vi "main OP600_V2.vi"() -> ()   [LabVIEW 2020]
uses:
  SubVI/OP600ZP_state.ctl
  <userlib>/Alex.vi/FGV.ctl
  VG/VG_progressBar.vi
  SubVI/CheminDeBase.vi
  VG/PN.vi
  VG/PackType.vi
  VG/IS30%.vi
  SubVI/OP600ZP_VGConf.vi
  VG/Ubatt.vi
  VG/OCV.vi
panel:
  out "Revision":i32
  out "Progres":dbl(slide) scale=0.0..30.0
  out "IS30% ?":bool
  out "Cluster":T1
  out "VISA OUT":T2
  out "progression":u8(slide) scale=0.0..100.0
  out "PN":string
  out "errout 2":errorcluster={"status"=TRUE, "code"=0, "source"="PCAN_CHANNEL ILLEGAL"} caption="errout"
  out "errout":errorcluster caption="sortie d'erreur"
  out "STOP":bool
  out "TOP":string
  out "DRAW":picture
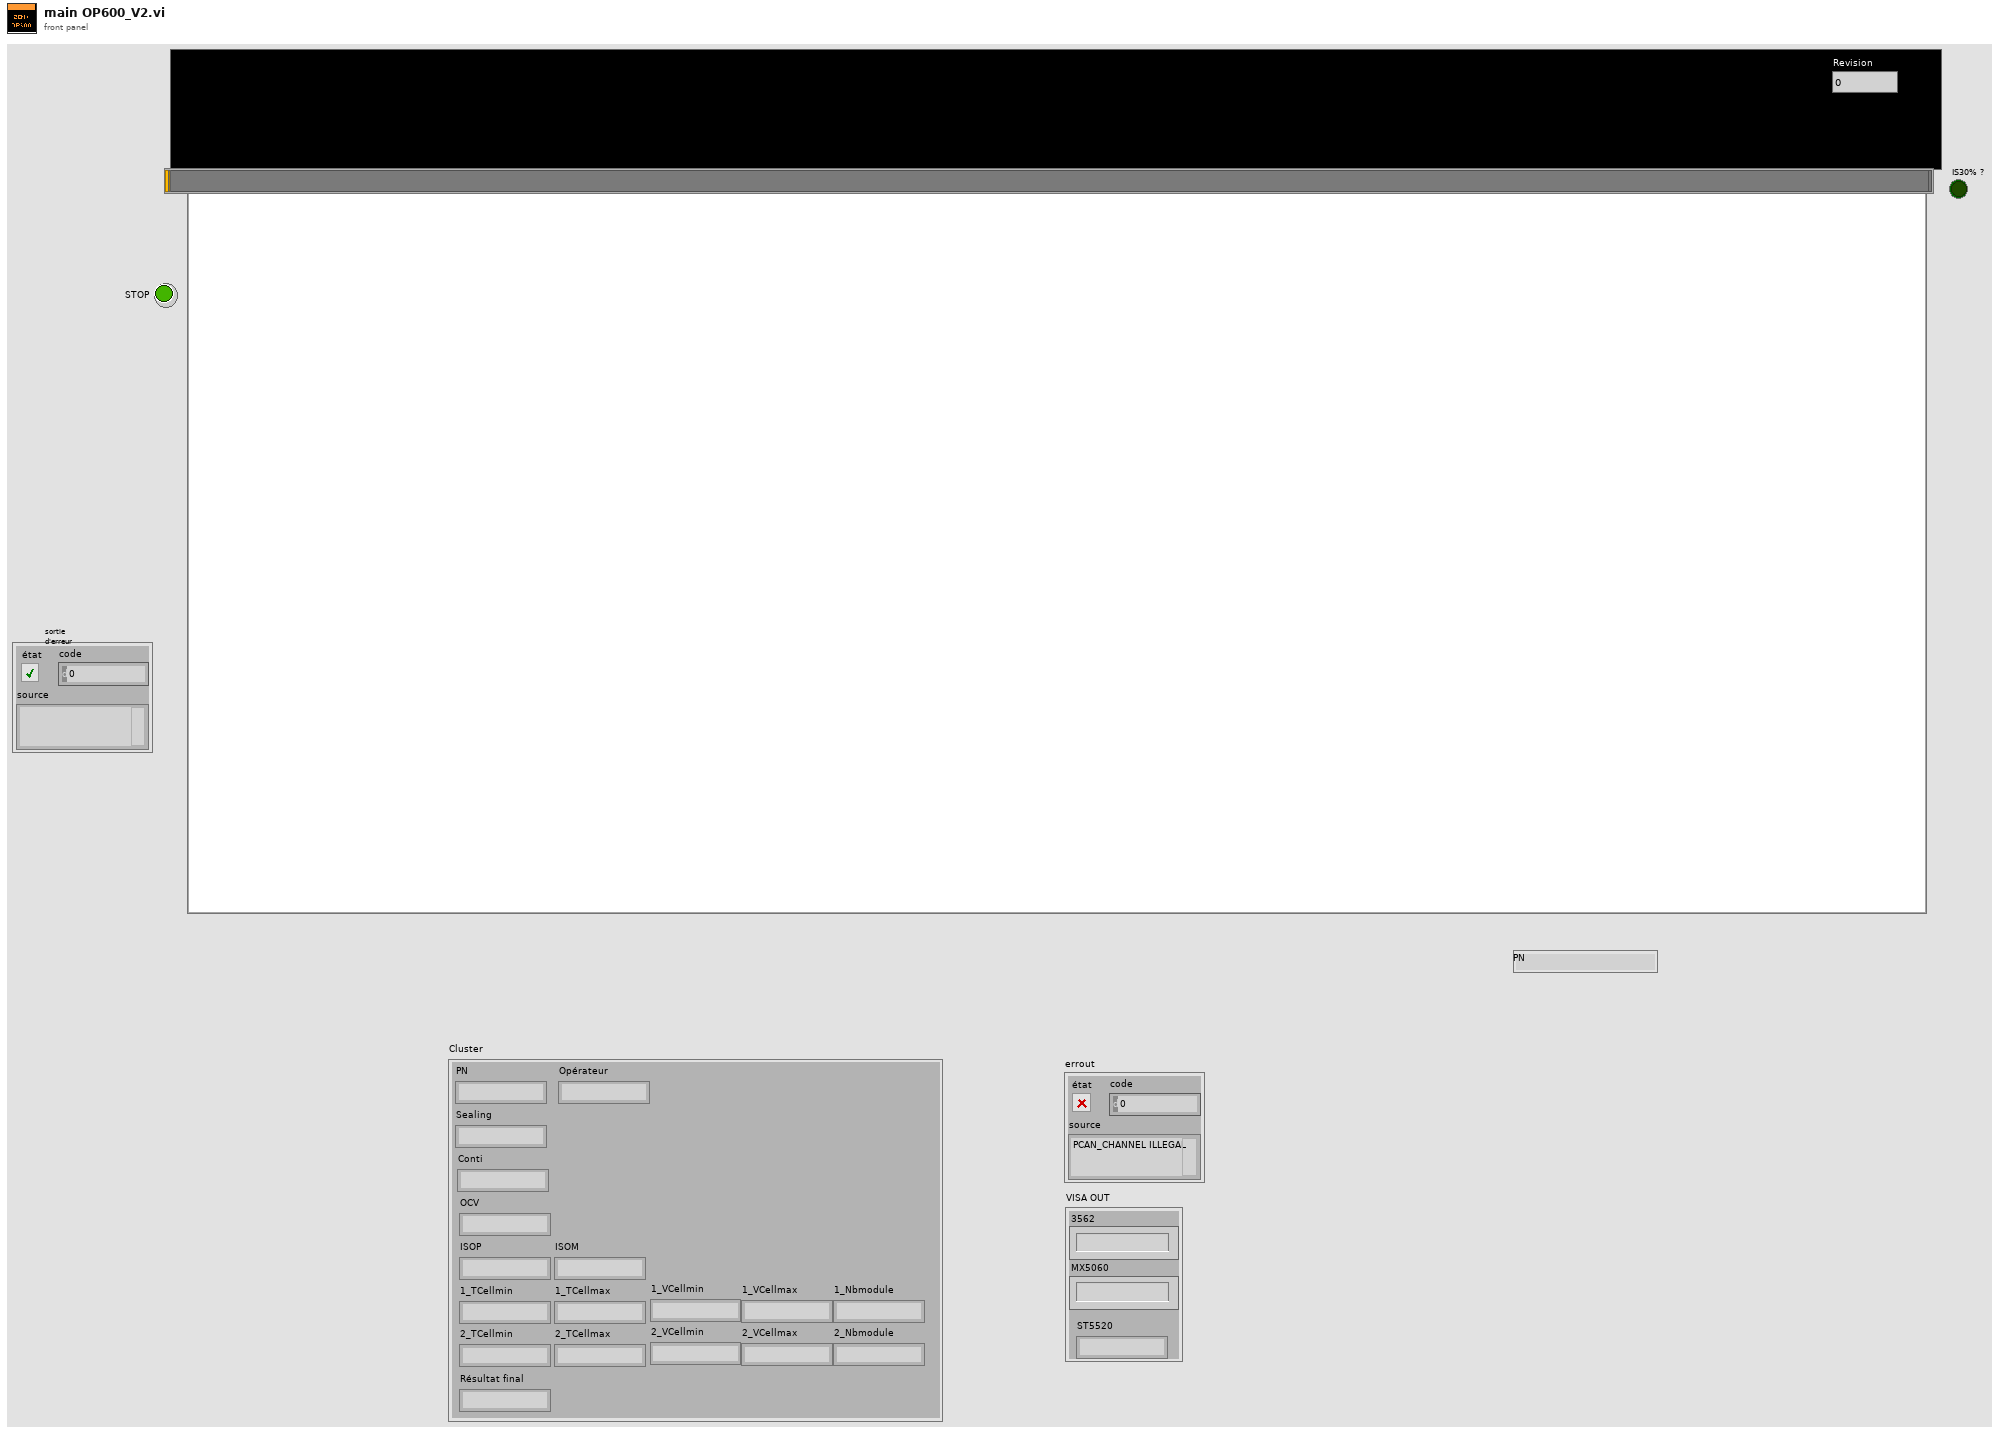
[diagram p1: front panel]
types:
  T1 = cluster{"PN":string, "Opérateur":string, "Sealing":string, "Conti":string, "OCV":string, "ISOP":string, "ISOM":string, "1_TCellmin":string, "1_TCellmax":string, "1_VCellmin":string, "1_VCellmax":string, "1_Nbmodule":string, "2_TCellmin":string, "2_TCellmax":string, "2_VCellmin":string, "2_VCellmax":string, "2_Nbmodule":string, "Résultat final":string}
  T2 = cluster{"3562":string, "MX5060":string, "ST5520":string}
  T3 = cluster{"PN":string, "Sealing":string, "Opérateur":string, "Conti":string, "OCV":string, "ISOP":string, "ISOM":string, "1_TCellmin":string, "1_TCellmax":string, "1_VCellmin":string, "1_VCellmax":string, "1_Nbmodule":string, "2_TCellmin":string, "2_TCellmax":string, "2_VCellmin":string, "2_VCellmax":string, "2_Nbmodule":string, "Résultat final":string}
  T4 = typedef "OP600ZP_state.ctl" = enum16{"Null", "Demarrage", "Init", "Scan", "Sealing", "VAT", "Conti", "CAN Resistance", "Softs", "MCU", "Iso", "OCV", "DTC", "PreCharge", "DTC2", "PARK", "FIN_TEST", "PackVoltage", "Capacitance", "INTERLOOP", "Current + DCIR", "DataDyn", "Crash", "Next", "Comext"}
  T5 = typedef "FGV.ctl" = enum16{"GET", "SET", "RAZ"}
  T6 = cluster{"BatteryVoltage@30s":dbl, "BatteryCurrent@30s":dbl, "DeltaV@30s":dbl, "DeltaT@30s":dbl, " BatteryCurrent":dbl, "DeltaV@0s":dbl, "DeltaT@0s":dbl, "Post Relax Voltage :":dbl}
  T7 = typedef "imagedata.ctl" = cluster{"image type":i32, "image depth":i32, "image":u8[], "mask":u8[], "colors":u32[], "Rectangle":cluster{"left":i16, "top":i16, "right":i16, "bottom":i16}}
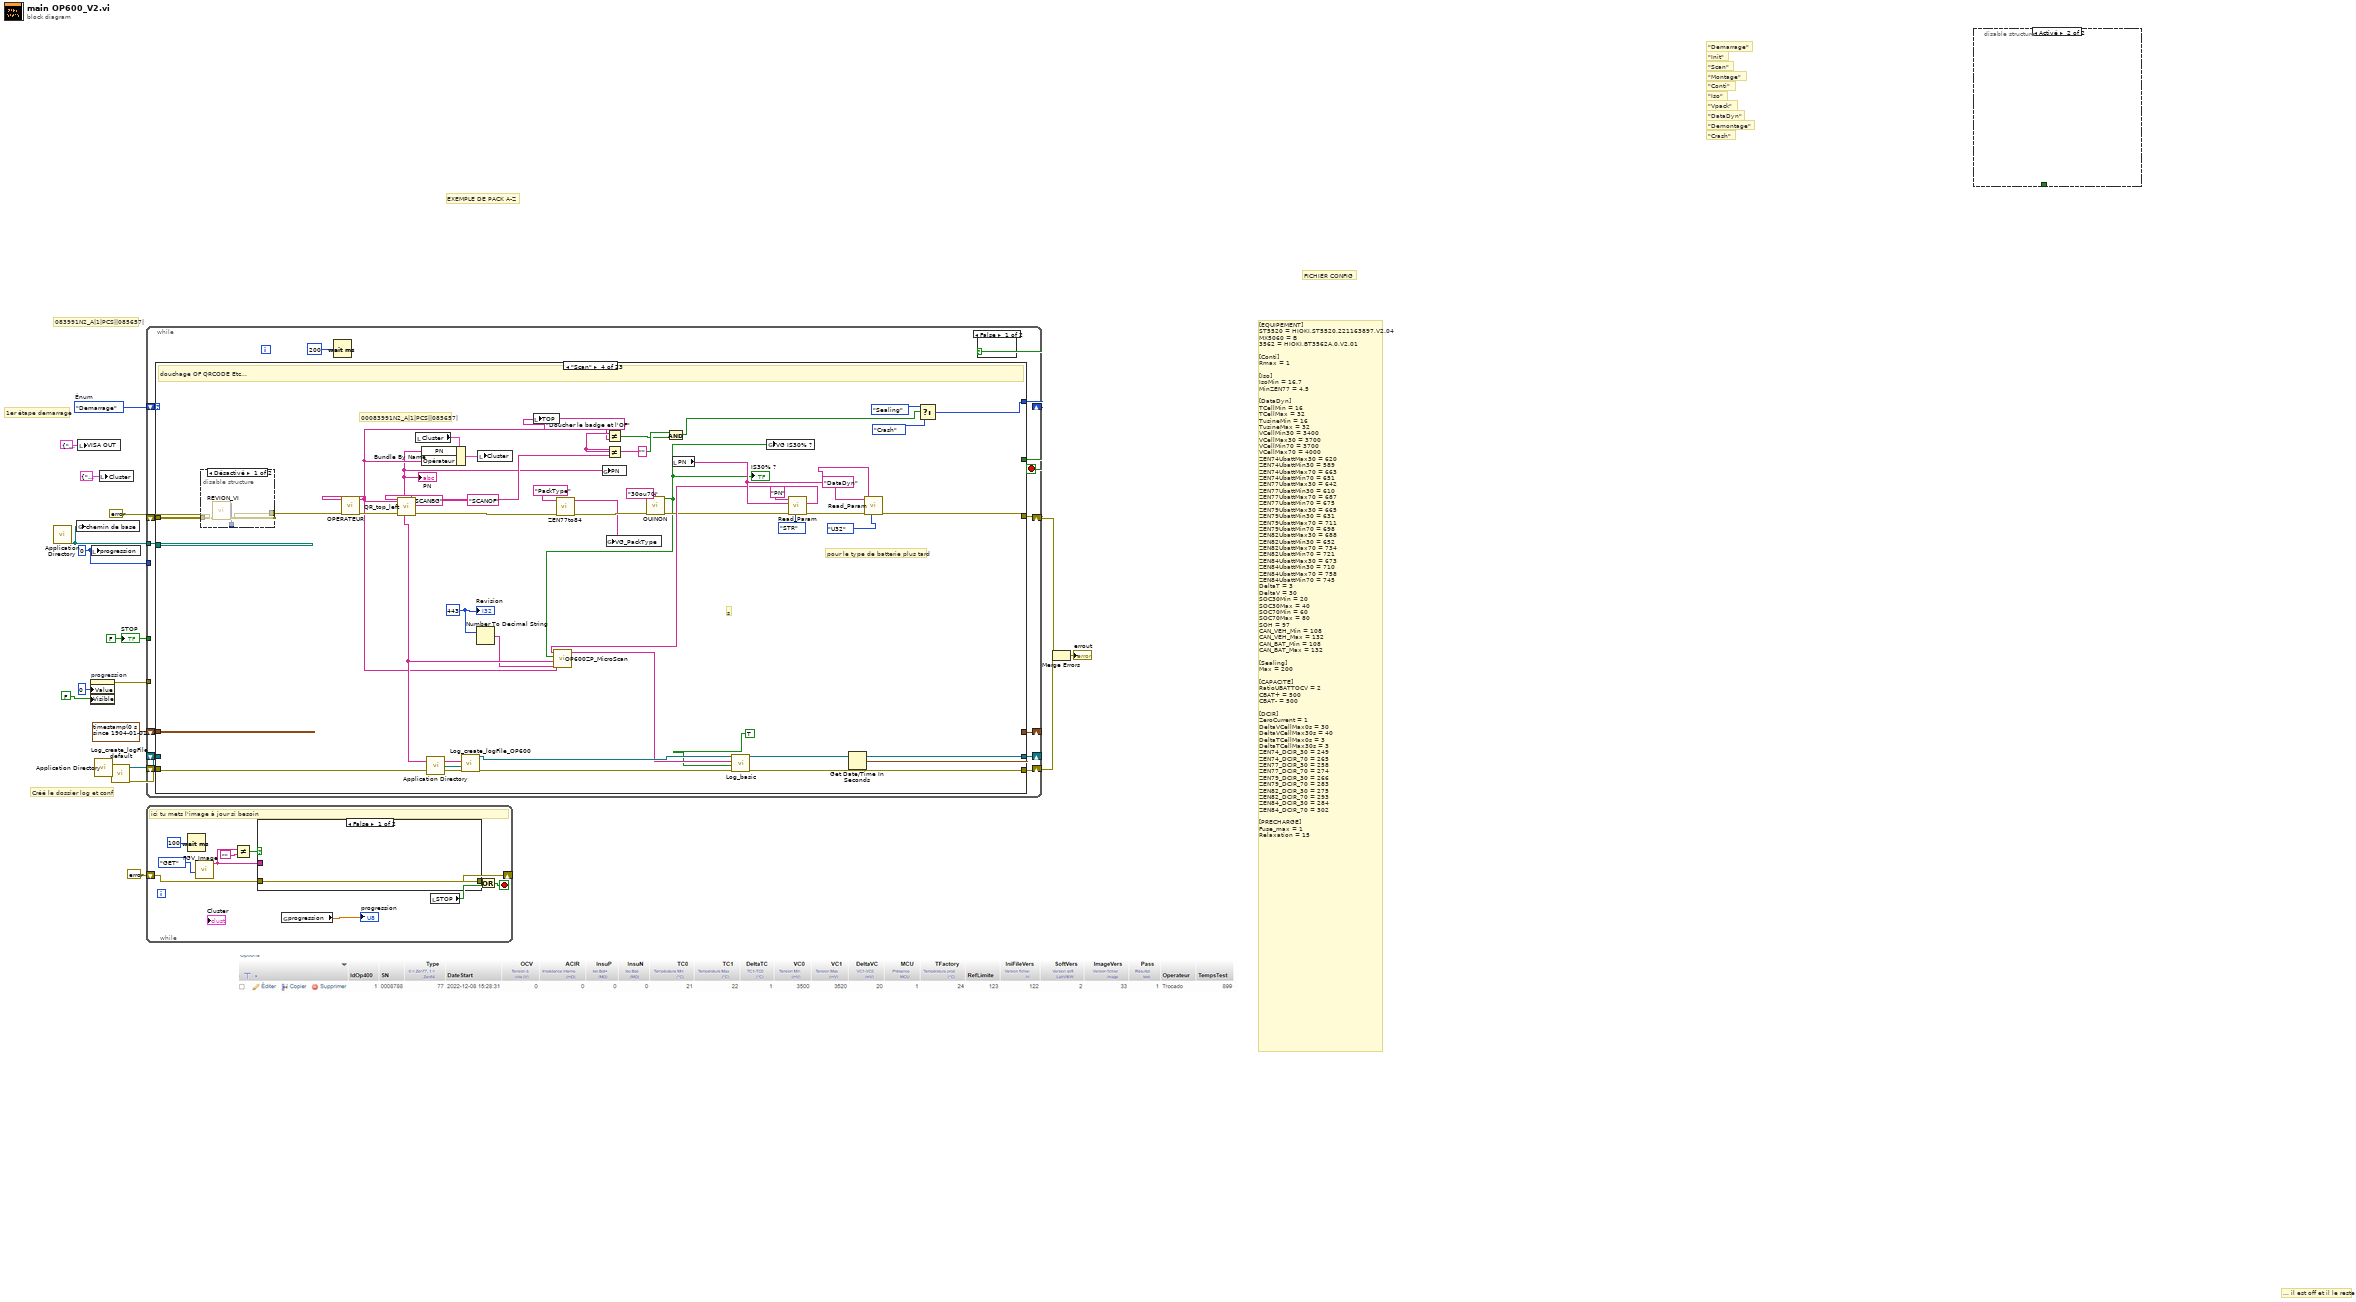
[diagram p0: block diagram]
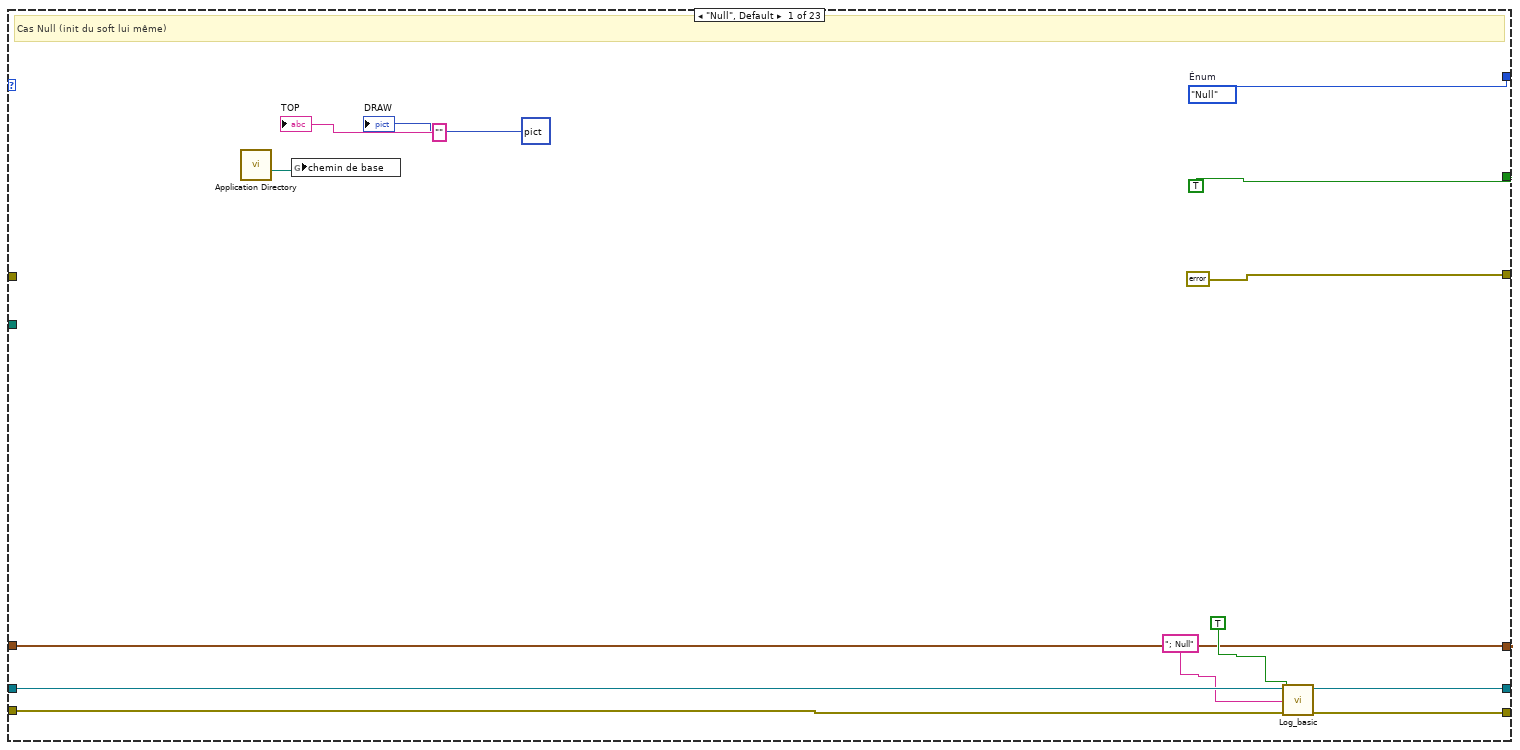
[diagram p2: hidden frame]
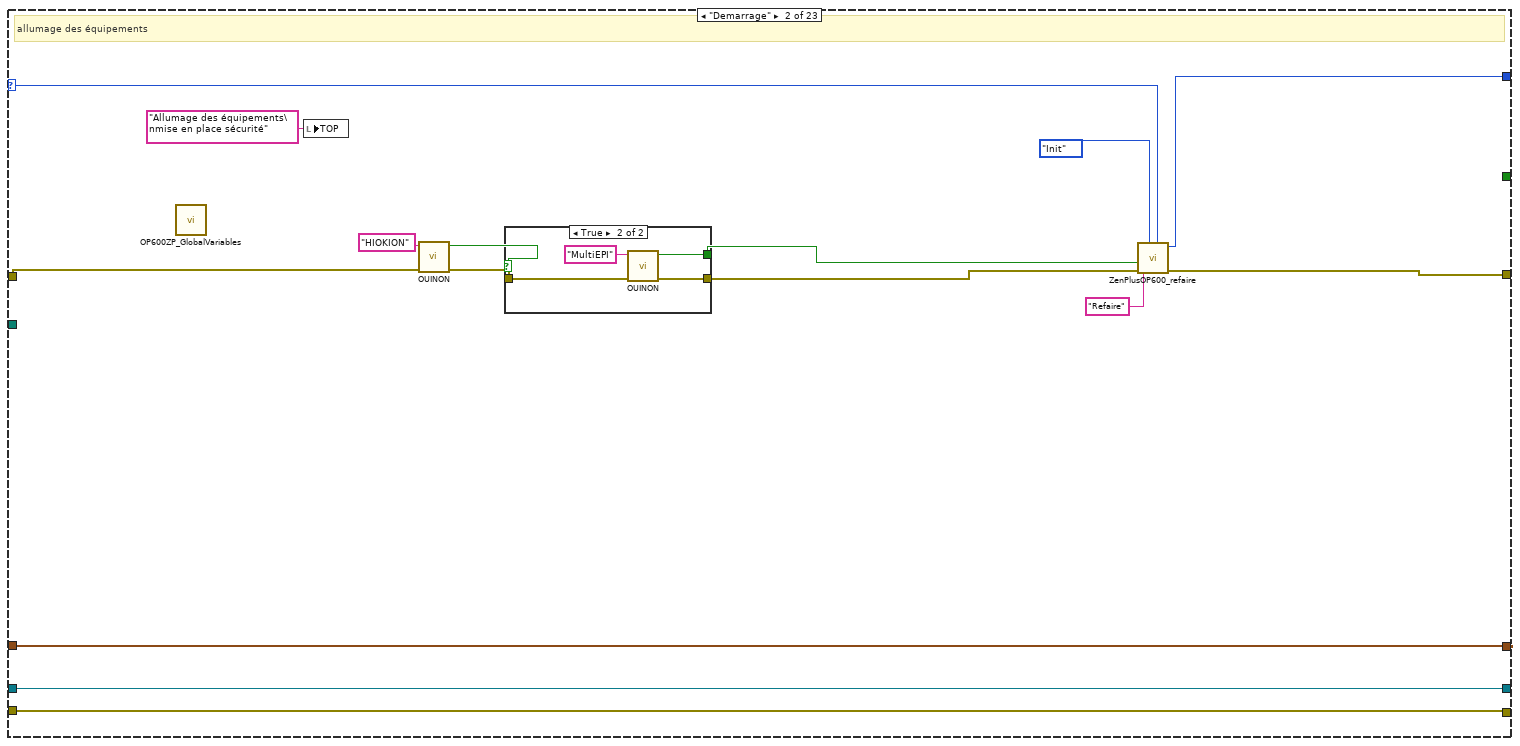
[diagram p3: hidden frame]
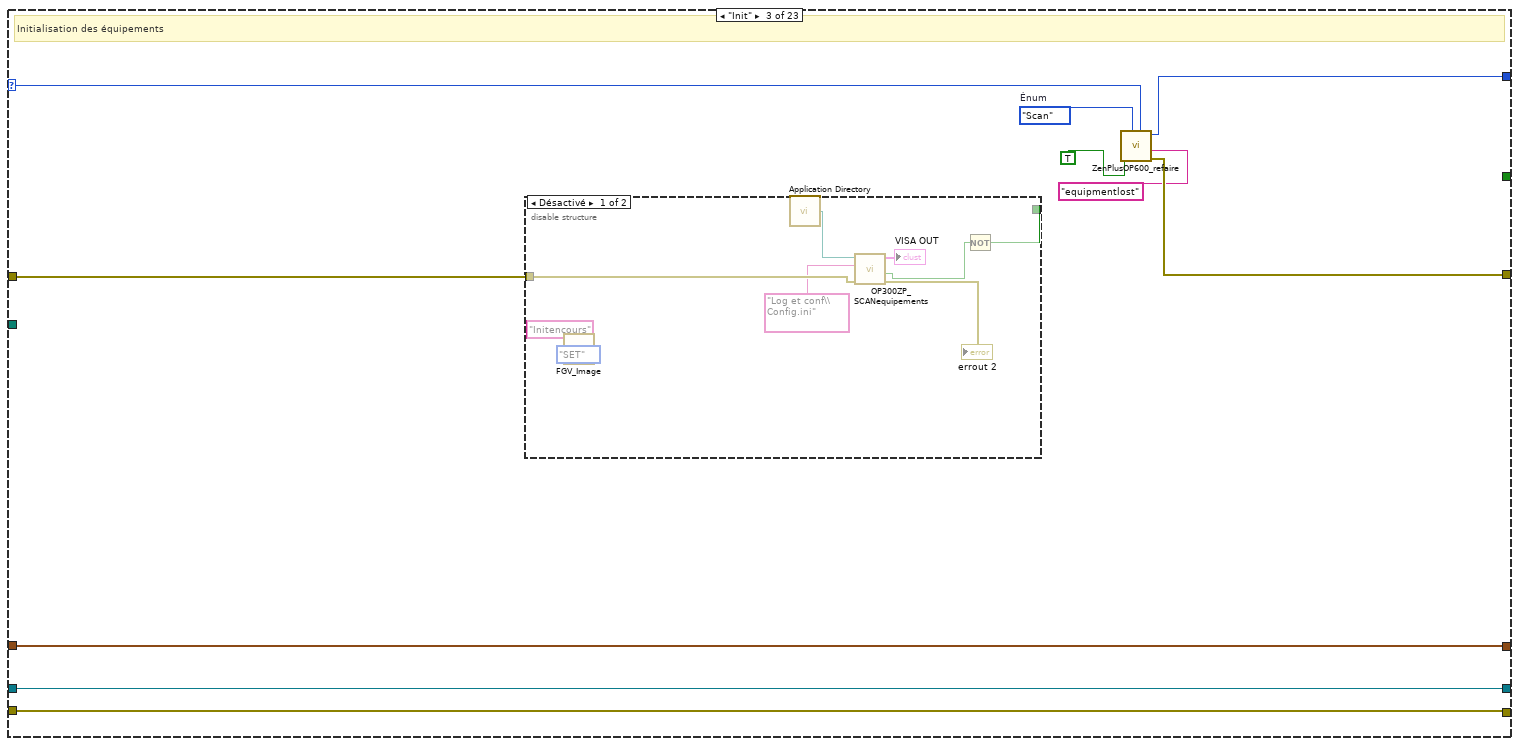
[diagram p5: hidden frame]
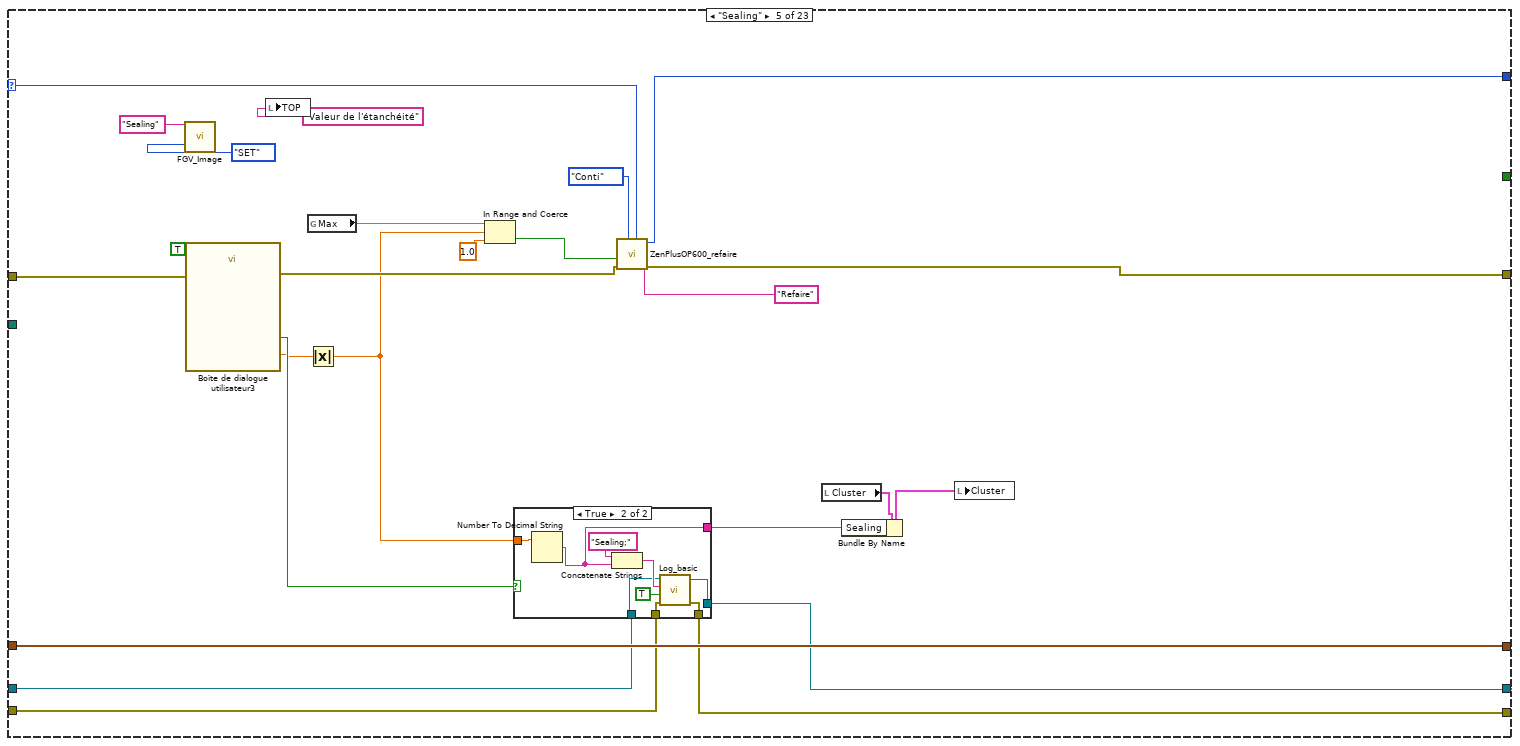
[diagram p8: hidden frame]
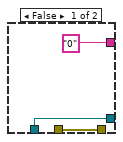
[diagram p9: hidden frame]
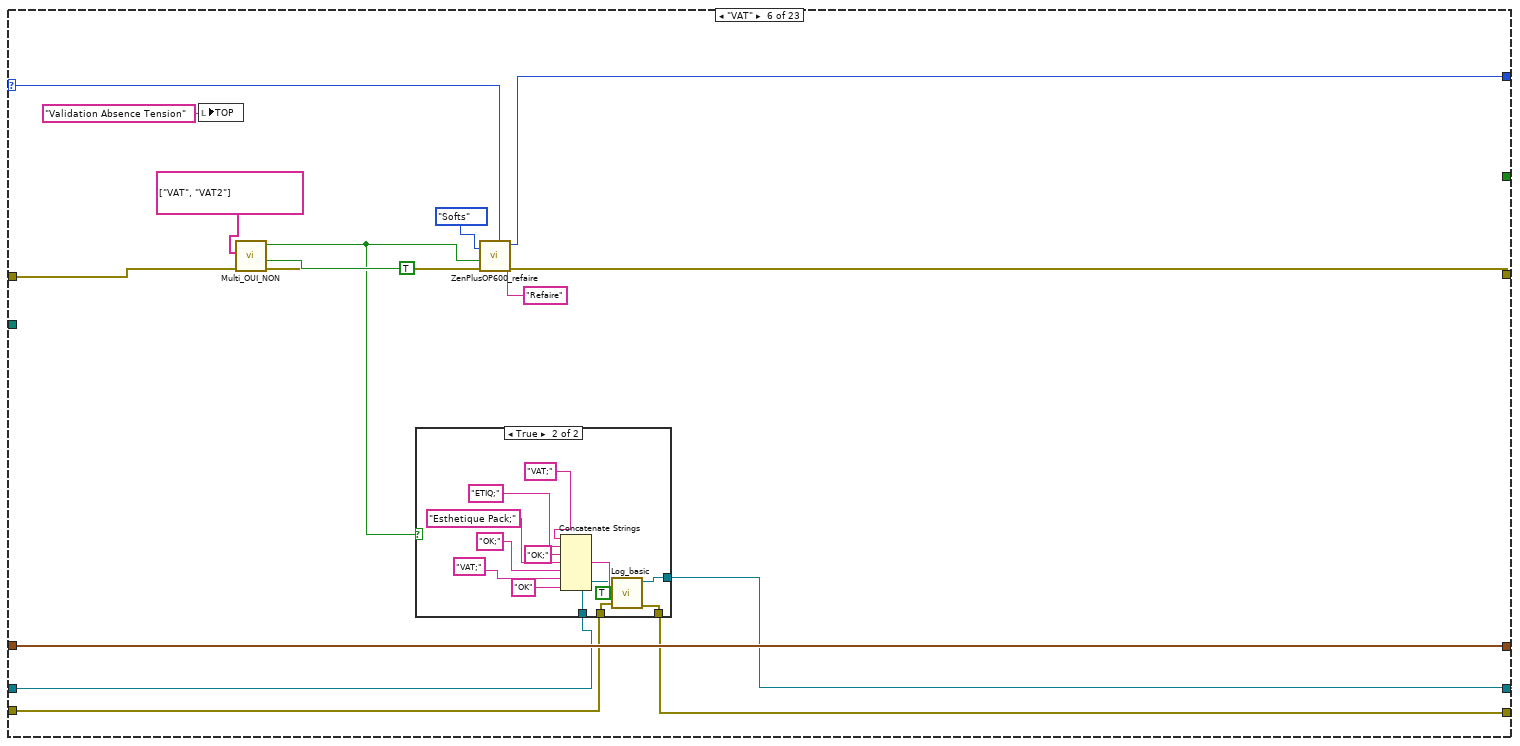
[diagram p10: hidden frame]
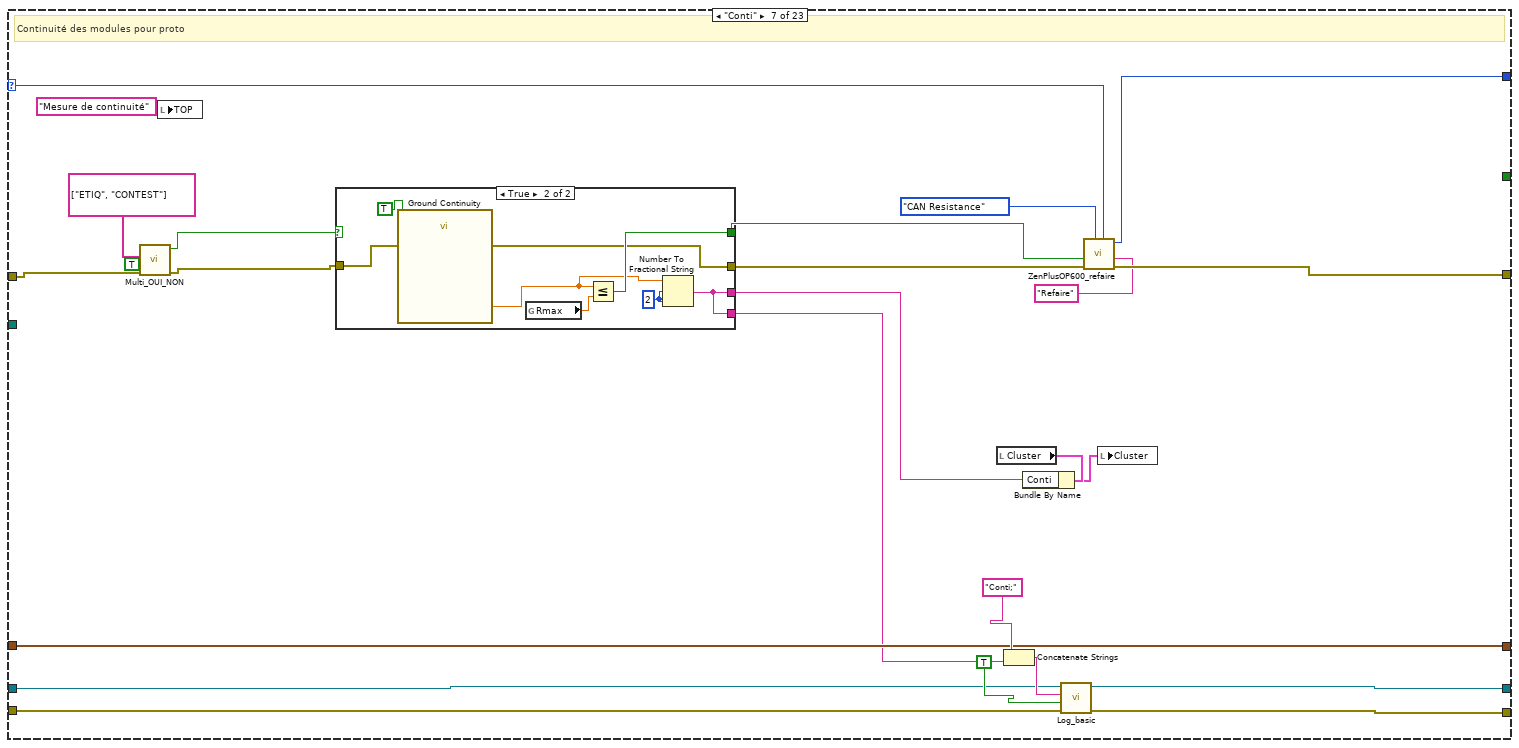
[diagram p12: hidden frame]
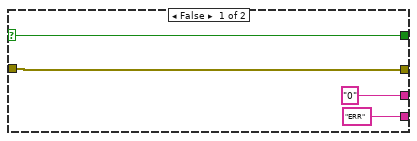
[diagram p13: hidden frame]
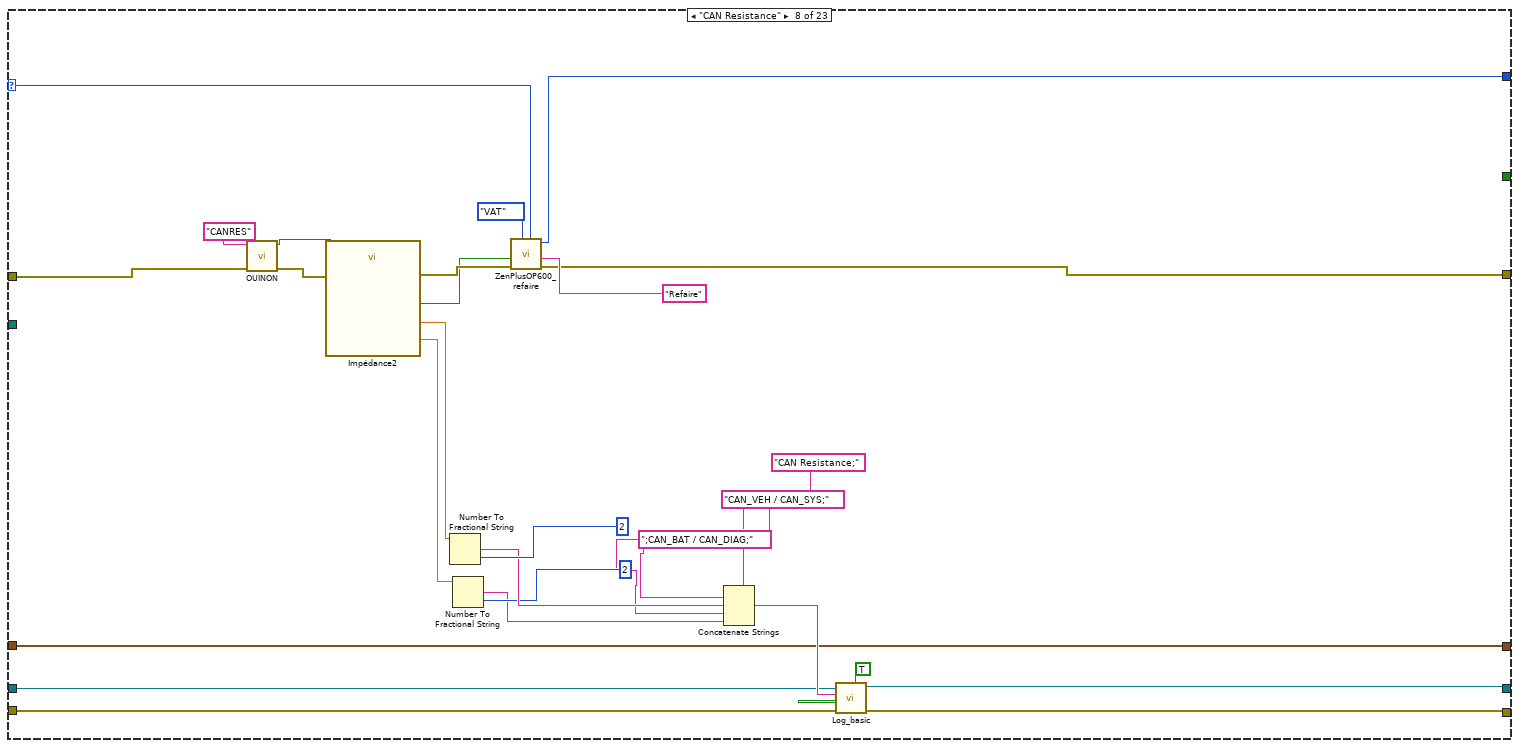
[diagram p14: hidden frame]
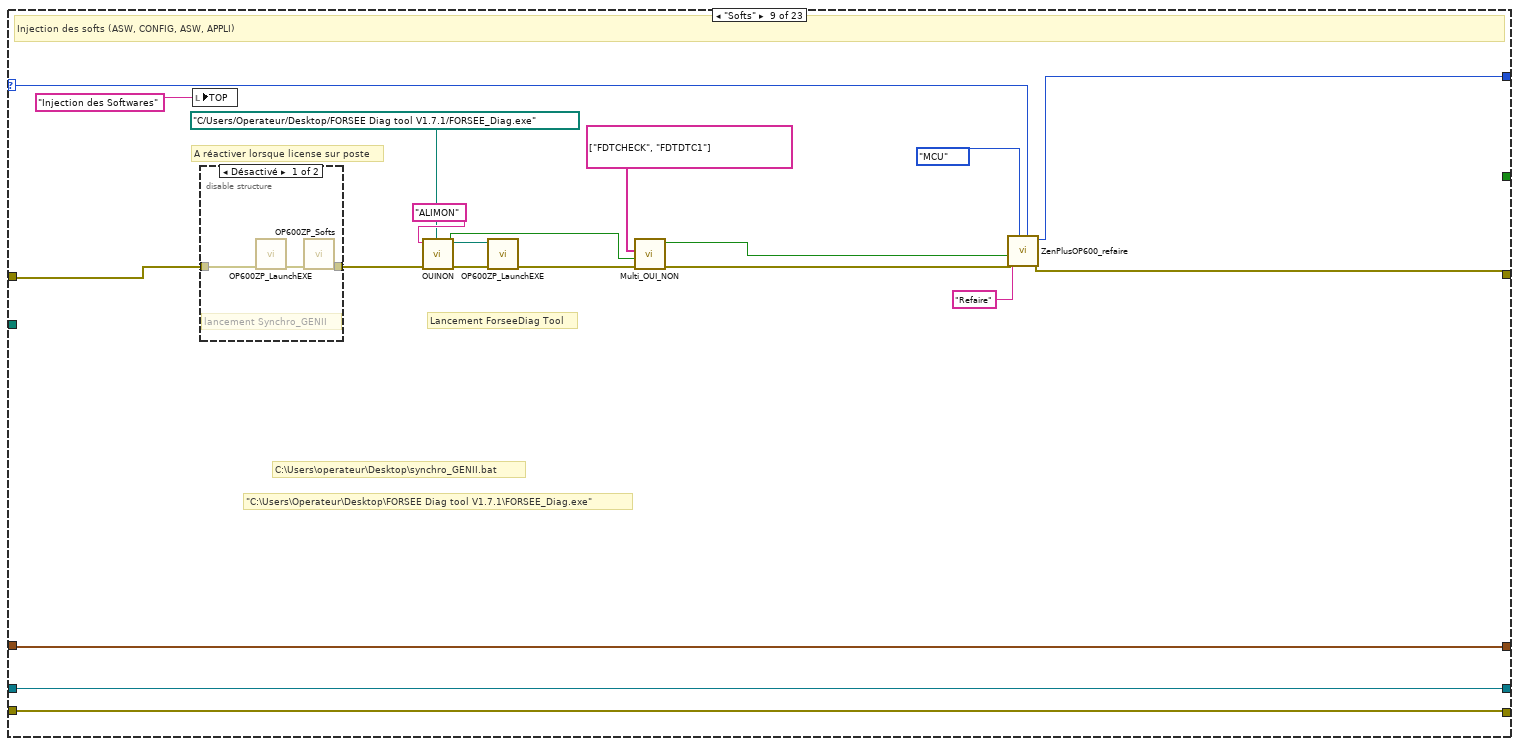
[diagram p15: hidden frame]
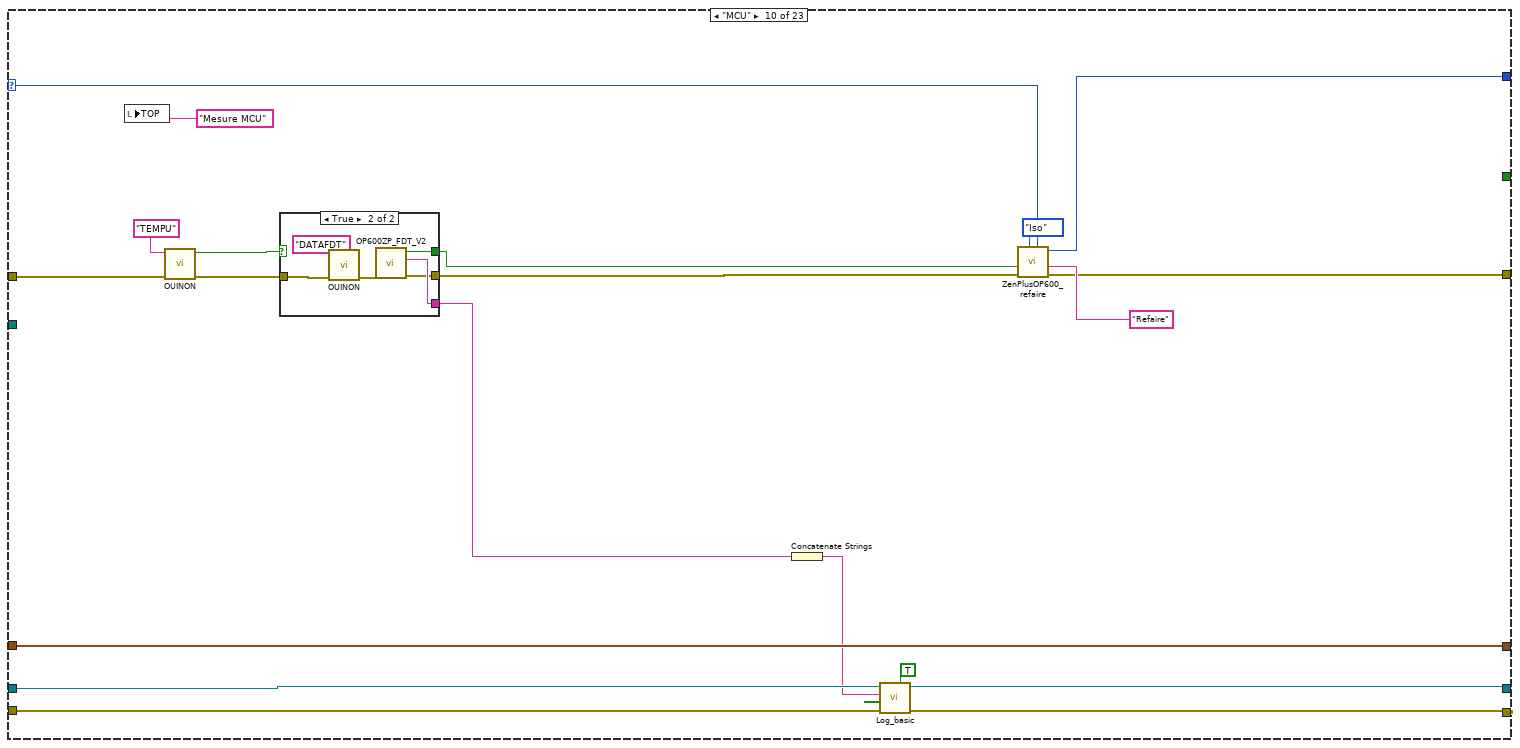
[diagram p17: hidden frame]
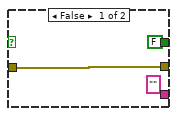
[diagram p18: hidden frame]
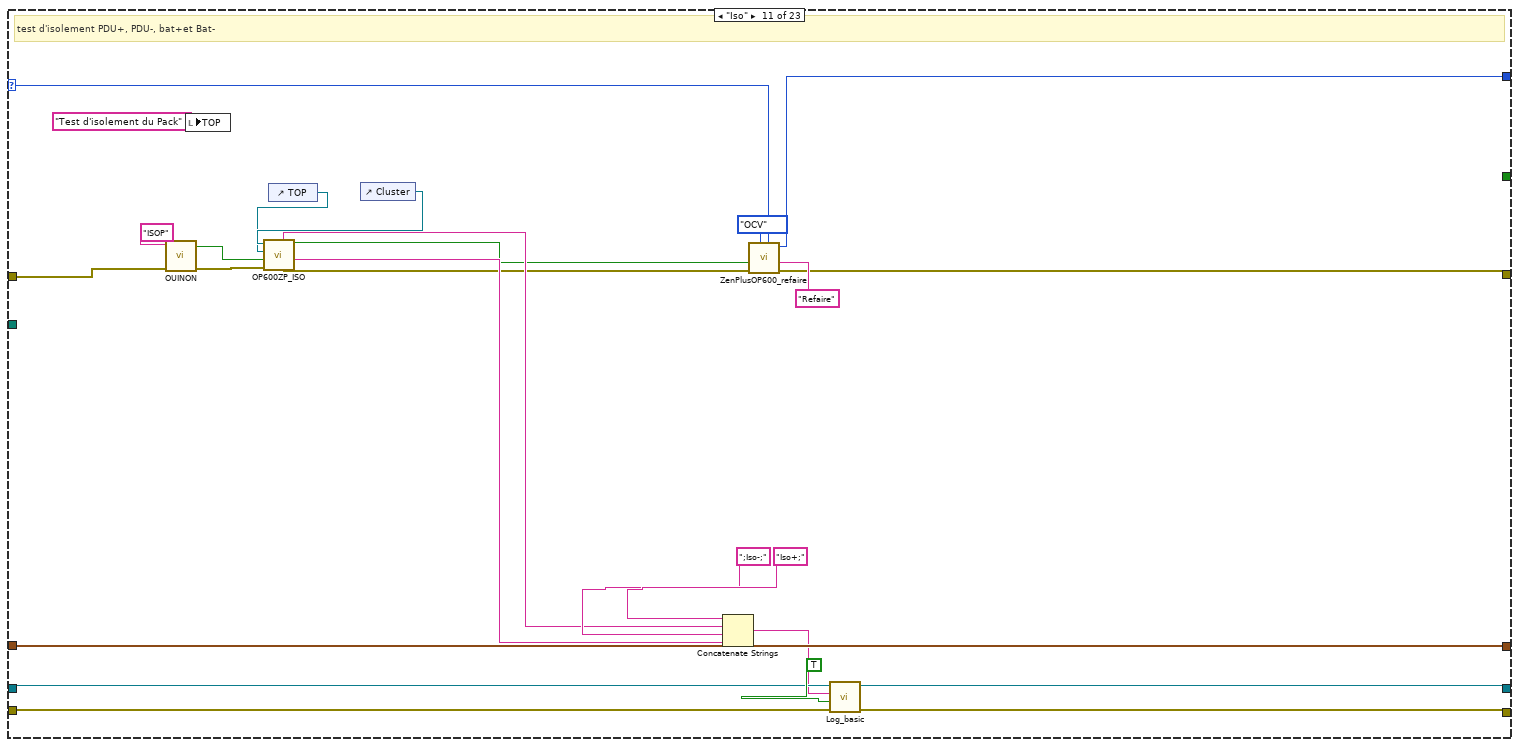
[diagram p19: hidden frame]
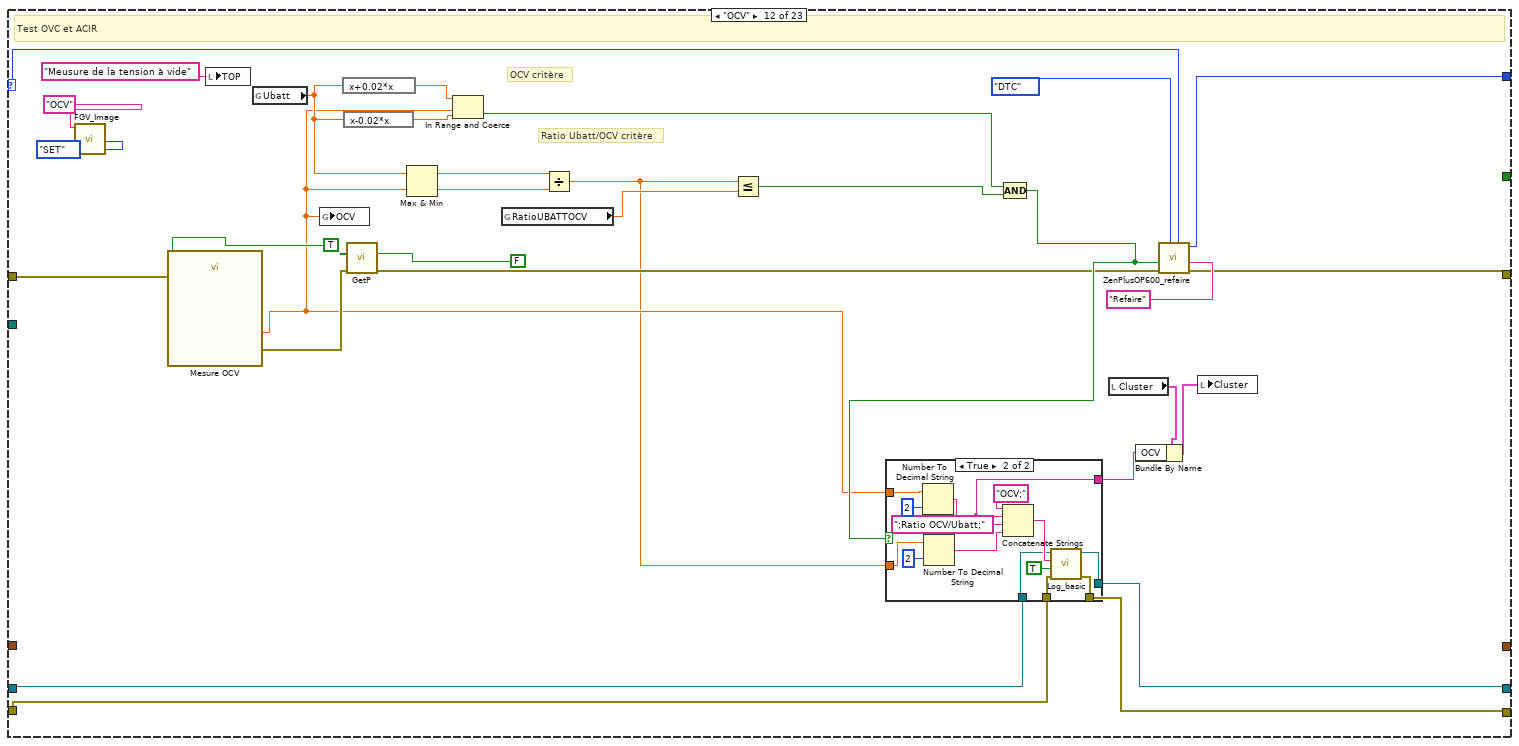
[diagram p20: hidden frame]
diagram:
  w8 = u8 0 ("progression")
  w1 = OP600ZP_state."Demarrage"  # Énum
  w14 = FALSE ("STOP")
  # "083991N2_A|1|PCS||085657|"
  # "[EQUIPEMENT]\nST5520 = HIOKI,ST5520,221163897,V2.04\t\nMX5060 = B\n3562 = HIOKI,BT3562A,0,V2.01\n\n[Conti]\nRmax = 1\n\n[Iso]\nIsoMin = 16.7\nMinZEN77 = 4.5\n\n[DataDyn]\nTCellMin = 16\nTCellMax = 32\nTusineMin = 16\nTusineMax = 32\nVCellMin30 = 3400\nVCellMax30 = 3700\nVCellMin70 = 3700\nVCellMax70 = 4000\nZEN74UbattMax30 = 620\nZEN74UbattMin30 = 589\nZEN74UbattMax70 = 663\nZEN74UbattMin70 = 651\nZEN77UbattMax30 = 642\nZEN77UbattMin30 = 610\nZEN77UbattMax70 = 687\nZEN77UbattMin70 = 675\nZEN79UbattMax30 = 665\nZEN79UbattMin30 = 631\nZEN79UbattMax70 = 711\nZEN79UbattMin70 = 698\nZEN82UbattMax30 = 688\nZEN82UbattMin30 = 652\nZEN82UbattMax70 = 734\nZEN82UbattMin70 = 721\nZEN84UbattMax30 = 673\nZEN84UbattMin30 = 710\nZEN84UbattMax70 = 758\nZEN84UbattMin70 = 745\nDeltaT = 3\nDeltaV = 30\nSOC30Min = 20\nSOC30Max = 40\nSOC70Min = 60\nSOC70Max = 80\nSOH = 97\nCAN_VEH_Min = 108\nCAN_VEH_Max = 132\nCAN_BAT_Min = 108\nCAN_BAT_Max = 132\n\n[Sealing]\nMax = 200\n\n[CAPACITE]\nRatioUBATTOCV = 2\nCBAT+ = 500\nCBAT- = 500\n\n[DCIR]\nZeroCurrent = 1\nDeltaVCellMax0s = 30\nDeltaVCellMax30s = 40\nDeltaTCellMax0s = 3\nDeltaTCellMax30s = 3\nZEN74_DCIR_30 = 249\nZEN74_DCIR_70 = 265\nZEN77_DCIR_30 = 258\nZEN77_DCIR_70 = 274\nZEN79_DCIR_30 = 266\nZEN79_DCIR_70 = 283\nZEN82_DCIR_30 = 275\nZEN82_DCIR_70 = 293\nZEN84_DCIR_30 = 284\nZEN84_DCIR_70 = 302\n\n[PRECHARGE]\nFuse_max = 1\nRelaxation = 15"
  # "EXEMPLE DE PACK A-Z"
  # "FICHIER CONFIG"
  # "Créé le dossier log et conf"
  # "1er étape demarrage"
  # "\"Crash\""
  # "\"Demontage\""
  # "\"DataDyn\""
  # "\"Iso\""
  # "\"Montage\""
  # "\"Scan\""
  # "\"Init\""
  # "\"Demarrage\""
  # "\"Conti\""
  # "\"Vpack\""
  # "... il est off et il le reste"
  n1 = call <vilib>:"Application Directory.vi"() -> ("Application Directory"=w13:path)
  n2 = global write "CheminDeBase.vi" "chemin de base"(w13) -> ()
  n3 = local write "VISA OUT"(T2 {"3562"="", "MX5060"="", "ST5520"=""} ("VISA OUT")) -> ()
  n4 = property on="progression" class="Slide (strict)"("Value"=u8 0 ("progression"), "Visible"=FALSE) -> (error out=w6:errorcluster)  [unwired: 2 in, 1 out]
  n5 = local write "progression"(w8) -> ()
  n6 = call <vilib>:"Application Directory.vi"() -> ("Application Directory"=w11:path)
  n7 = local write "Cluster"(T3 {"PN"="0", "Sealing"="0", "Opérateur"="0", "Conti"="0", "OCV"="0", "ISOP"="0", "ISOM"="0", "1_TCellmin"="0", "1_TCellmax"="0", "1_VCellmin"="0", "1_VCellmax"="0", "1_Nbmodule"="0", "2_TCellmin"="0", "2_TCellmax"="0", "2_VCellmin"="0", "2_VCellmax"="0", "2_Nbmodule"="0", "Résultat final"="0"} ("Cluster")) -> ()
  n8 = call <userlib>:"Log_create_logFile_default.vi"("appdir"=w11) -> ("errout"=w12:errorcluster, "Fichier à flux d'octets en sortie"=w15:refnum<file>)  [unwired: 9 in]
  n9 = while {
    shift-right: [w30] -> w17
    shift-left: errorcluster {"status"=FALSE, "code"=0, "source"=""} ("error out") -> [w21]
    shift-right: [w26] -> w16
    shift-left: w12 -> [w29]
    shift-right: [w27] -> _
    shift-left: w15 -> [w28]
    tunnel: w13 -> [w24]
    tunnel: w14 -> [_]
    shift-right: [w22] -> _
    shift-left: timestamp(0 s since 1904-01-01) ("seconds since 1Jan1904") -> [w23]
    tunnel: w8 -> [_]
    tunnel: w6 -> [_]
    shift-right: [w19] -> _
    shift-left: w1 -> [w20]
    stop <- w25 stop-if-true
    n10 = case shown="\"Scan\"" w20 {
      selector: w20 -> [_ w46 w68 _ w141 w177 w207 w242 w273 w291 w319 w346 w393 w460 w523 w569 w644 w698 w759 w774 _ _ w867]
      tunnel: w21 -> [_ w58 w72 w88 w157 w183 w205 w263 w266 w294 w320 w364 w400 w483 w508 w577 w665 w697 w750 w772 w821 w858 w864]
      tunnel: [errorcluster {"status"=FALSE, "code"=0, "source"=""} ("errin") w49 w71 w111 w137 w175 w216 w239 w275 w299 w324 w363 w411 w461 w521 w570 w645 w689 _ _ w821 w830 w866] -> w30
      tunnel: w29 -> [w40 w52 w75 w126 w148 w173 w223 w248 w281 w306 w339 w360 w406 w475 w529 w564 w648 w695 w757 w771 w824 w855 w870]
      tunnel: w28 -> [w41 w59 w74 _ w149 w171 w222 w246 w280 w305 w338 w362 w404 w473 w530 w562 w651 w696 w756 w768 w825 w856 w869]
      tunnel: [w38 w59 w74 w128 w146 w170 w221 w245 w280 w303 w337 w361 w403 w472 w527 w561 w650 w693 w753 w769 _ _ w861] -> w27
      tunnel: [w39 w52 w75 w129 w147 w172 w220 w247 w281 w304 w340 w359 w405 w474 w528 w563 w649 w692 w754 w770 w798 w829 w868] -> w26
      tunnel: [TRUE _ _ _ _ _ _ _ _ _ _ _ _ _ _ _ _ _ _ _ w826 _ _] -> w25
      tunnel: w24 -> [_ _ _ _ _ _ _ _ _ _ _ _ _ _ _ _ _ _ _ _ _ _ w865]
      tunnel: w23 -> [w35 w57 w73 _ w150 w179 w218 w244 w283 w302 w336 _ w401 w470 w526 w567 w666 w694 w755 _ _ _ w862]
      tunnel: [w35 w57 w73 w118 w150 w179 w218 w244 w283 w302 w336 _ w401 w470 w526 w567 w666 w694 w755 _ _ _ w863] -> w22
      tunnel: [w32 w45 w66 w89 w140 w176 w206 w240 w271 w289 w317 w344 w391 w458 w522 w566 w643 w691 w758 w773 OP600ZP_state."Crash" w828 w860] -> w19
      frame "Null", Default {
        w32 = OP600ZP_state."Null"  # Énum
        # "Cas Null (init du soft lui même)"
        n11 = call <vilib>:"Application Directory.vi"() -> ("Application Directory"=w44:path)
        n12 = global write "CheminDeBase.vi" "chemin de base"(w44) -> ()
        n13 = call <userlib>:"Log_basic.vi"("errin"=w40, "date?"=TRUE, "chaîne"="; Null", "in"=w41) -> ("sortie d'erreur"=w39:errorcluster, "refnum en sortie"=w38:refnum<file>)  [unwired: 6 in]
        "DRAW" <- picture data[5B] ("DRAW")
        "TOP" <- "" ("TOP")
      }
      frame "Demarrage" {
        # "allumage des équipements"
        n14 = call "OP600ZP_GlobalVariables.vi"() -> ()  [unwired: 12 in]
        n15 = local write "TOP"("Allumage des équipements\nmise en place sécurité" ("TOP")) -> ()
        n16 = call "OUINON.vi"("errin"=w58, "image"="HIOKION") -> ("error out"=w53:errorcluster, "OUI/NON"=w54:bool)  [unwired: 8 in]
        n17 = case shown="True" w54 {
          selector: w54 -> [w61 _]
          tunnel: [w61 w65] -> w48
          tunnel: [w60 w64] -> w50
          tunnel: w53 -> [w60 w62]
          frame False {
          }
          frame True {
            n18 = call "OUINON.vi"("errin"=w62, "image"="MultiEPI" ("IN")) -> ("error out"=w64:errorcluster, "OUI/NON"=w65:bool)  [unwired: 8 in]
          }
        }
        n19 = call "ZenPlusOP600_refaire.vi"("image"="Refaire", "Refaire"=w46, "Cas ok"=OP600ZP_state."Init" ("casOK"), "errin"=w50, "test ok ?"=w48) -> ("errout"=w49:errorcluster, "Next"=w45:T4)  [unwired: 5 in]
      }
      frame "Init" {
        w67 = OP600ZP_state."Scan"  # Énum
        # "Initialisation des équipements"
        n20 = disable-structure shown="Désactivé" {
          disable-tunnel: w72 -> [w84 _]
          disable-tunnel: [w79 _] -> _
          frame Disabled {
            n21 = call <userlib>:"FGV_Image.vi"("Énum"=FGV."SET", "IN"="Initencours") -> ()  [unwired: 9 in, 1 out]
            n22 = call <vilib>:"Application Directory.vi"() -> ("Application Directory"=w80:path)
            n23 = call "OP300ZP_SCANequipements.vi"("Errin"=w84, "Chaîne"="Log et conf\\Config.ini", "pathin"=w80) -> ("errout"=→"errout 2":errorcluster, "KO?"=w78:bool, "VISA OUT"=→"VISA OUT":T2)  [unwired: 6 in]
            n24 = Not(x=w78) -> (.not. x?=w79:bool)
          }
          frame Enabled {
          }
        }
        n25 = call "ZenPlusOP600_refaire.vi"("image"="equipmentlost", "Refaire"=w68, "Cas ok"=w67, "test ok ?"=TRUE) -> ("errout"=w71:errorcluster, "Next"=w66:T4)  [unwired: 6 in]
      }
      frame "Scan" {
        w86 = 443
        w121 = "" ("x")
        # "s"
        # "pour le type de batterie plus tard"
        # "00083991N2_A|1|PCS||085657|"
        # "douchage OF QRCODE Etc..."
        n26 = disable-structure shown="Désactivé" {
          disable-tunnel: w88 -> [w132 _]
          disable-tunnel: [w131 _] -> w87
          disable-tunnel: [w130 _] -> _
          frame Disabled {
            n27 = call "REVION_VI.vi"("ERRIN"=w132) -> ("ERROUT"=w131:errorcluster, "N° Révision"=w130:u32)  [unwired: 9 in]
          }
          frame Enabled {
          }
        }
        n28 = call <userlib>:"OPERATEUR.vi"("errin"=w87, "IN"="SCANBG") -> ("error out"=w117:errorcluster, "Dataout"=w98:string)  [unwired: 8 in]
        n29 = call "QR_top_left.vi"("errin"=w117, "image"="SCANOF") -> ("error out"=w93:errorcluster, "Réponse"=w115:string, "SN"=w114:string, "PN"=w94:string)  [unwired: 5 in, 1 out]
        "PN" <- w94
        n30 = local read "Cluster"() -> (w100:T1)
        n31 = Bundle By Name(cluster=w100, "PN"=w94, "Opérateur"=w98) -> (w99:T1)
        n32 = call <vilib>:"Application Directory.vi"() -> ("Application Directory"=w127:path)
        n33 = call "Log_create_logFile_OP600.vi"("errin"=w126, "toute l'expression"=w114, "Application Directory"=w127) -> ("sortie d'erreur"=w124:errorcluster, "Fichier à flux d'octets en sortie"=w125:refnum<file>)  [unwired: 7 in]
        n34 = Number To Decimal String(number=w86) -> (decimal integer string=w85:string)  [unwired: 1 in]
        n35 = local write "Cluster"(w99) -> ()
        n36 = local write "TOP"("Doucher le badge et l'OF" ("TOP")) -> ()
        n37 = call <userlib>:"ZEN77to84.vi"("errin"=w93, "image"="PackType") -> ("error out"=w92:errorcluster, "Réponse"=w90:string)  [unwired: 8 in]
        n38 = global write "PN.vi" "PN"(w94) -> ()
        n39 = Not Equal?(x=w121, y=w98) -> (x != y?=w119:bool)
        n40 = Not Equal?(x=w121, y=w115) -> (x != y?=w120:bool)
        n41 = global write "PackType.vi" "VG_PackType"(w90) -> ()
        n42 = call "OUINON.vi"("errin"=w92, "image"="30ou70") -> ("error out"=w96:errorcluster, "OUI/NON"=w95:bool)  [unwired: 8 in]
        "IS30% ?" <- w95
        n43 = Compound Arithmetic op=AND ("Opérateur arithmétique")(w120, w119) -> (w104:bool)
        n44 = local read "PN"() -> (w107:string)
        n45 = global write "IS30%.vi" "VG IS30% ?"(w95) -> ()
        n46 = call <userlib>:"Read_Param.vi"("Énum"=enum16{"STR", "DBL", "U32"}."STR", "errin"=w96, "section"=w107, "key"="PN") -> ("error out"=w110:errorcluster, "str"=w106:string)  [unwired: 3 in, 3 out]
        n47 = call "OP600ZP_MicroScan.vi"("Dataout"=w98, "Rev"=w85, "SN"=w114, "Oui"=w95, "str"=w106) -> ("Chaîne"=w123:string)  [unwired: 6 in]
        n48 = call <userlib>:"Log_basic.vi"("errin"=w124, "date?"=TRUE, "chaîne"=w123, "in"=w125) -> ("sortie d'erreur"=w129:errorcluster, "refnum en sortie"=w128:refnum<file>)  [unwired: 6 in]
        n49 = Get Date/Time In Seconds() -> (seconds since 1Jan1904=w118:timestamp)
        n50 = call <userlib>:"Read_Param.vi"("Énum"=enum16{"STR", "DBL", "U32"}."U32", "errin"=w110, "section"="DataDyn", "key"=w107) -> ("error out"=w111:errorcluster)  [unwired: 3 in, 4 out]
        n51 = Select ("Sélectionner")(t=OP600ZP_state."Sealing" ("Énum"), s=w104, f=OP600ZP_state."Crash" ("cas faux")) -> (s? t:f=w89:T4)
        "Revision" <- w86
      }
      frame "Sealing" {
        n52 = call <userlib>:"FGV_Image.vi"("Énum"=FGV."SET", "IN"="Sealing") -> ()  [unwired: 9 in, 1 out]
        n53 = call "Boîte de dialogue utilisateur3"("Enable"=TRUE, "error in (no error)"=w157) -> ("Étenchéité"=w134:dbl, "OK"=w136:bool, "error out"=w138:errorcluster)  [unwired: 15 in]
        n54 = local write "TOP"("Valeur de l'étanchéité" ("TOP")) -> ()
        n55 = global read "OP600ZP_VGConf.vi" "Max"() -> (w139:dbl)
        n56 = Absolute Value(x=w134) -> (abs(x)=w133:dbl)
        n57 = In Range and Coerce(upper limit=w139, x=w133, lower limit=1.0 ("limite inférieure")) -> (In Range?=w154:bool)  [unwired: 1 out]
        n58 = case shown="True" w136 {
          tunnel: [w158 w166] -> w146
          tunnel: w133 -> [_ w165]
          tunnel: ["0" w164] -> w151
          tunnel: w149 -> [w158 w163]
          tunnel: w148 -> [w159 w162]
          tunnel: [w159 w161] -> w147
          frame False {
          }
          frame True {
            n59 = Number To Decimal String(number=w165) -> (decimal integer string=w164:string)  [unwired: 1 in]
            n60 = Concatenate Strings("Sealing;" ("chaîne"), w164) -> (w168:string)
            n61 = call <userlib>:"Log_basic.vi"("errin"=w162, "date?"=TRUE, "chaîne"=w168, "in"=w163) -> ("sortie d'erreur"=w161:errorcluster, "refnum en sortie"=w166:refnum<file>)  [unwired: 6 in]
          }
        }
        n62 = call "ZenPlusOP600_refaire.vi"("image"="Refaire", "Refaire"=w141, "Cas ok"=OP600ZP_state."Conti", "errin"=w138, "test ok ?"=w154) -> ("errout"=w137:errorcluster, "Next"=w140:T4)  [unwired: 5 in]
        n63 = local read "Cluster"() -> (w153:T1)
        n64 = Bundle By Name(cluster=w153, "Sealing"=w151) -> (w152:T1)
        n65 = local write "Cluster"(w152) -> ()
      }
      frame "VAT" {
        n66 = local write "TOP"("Validation Absence Tension" ("TOP")) -> ()
        n67 = call "Multi_OUI_NON.vi"("errin"=w183, "errinb"=TRUE, "Tableau"=string[] ["VAT", "VAT2"]) -> ("errout"=w180:errorcluster, "isok?"=w174:bool)  [unwired: 7 in]
        n68 = case shown="True" w174 {
          tunnel: [w187 w198] -> w172
          tunnel: w173 -> [w187 w197]
          tunnel: [w186 w196] -> w170
          tunnel: w171 -> [w186 w195]
          frame False {
          }
          frame True {
            n69 = Concatenate Strings("VAT;" ("chaîne"), "ETIQ;" ("chaîne"), "OK;" ("chaîne"), "Esthetique Pack;" ("chaîne"), "OK;" ("chaîne"), "VAT;" ("chaîne"), "OK" ("chaîne")) -> (w199:string)
            n70 = call <userlib>:"Log_basic.vi"("errin"=w197, "date?"=TRUE, "chaîne"=w199, "in"=w195) -> ("sortie d'erreur"=w198:errorcluster, "refnum en sortie"=w196:refnum<file>)  [unwired: 6 in]
          }
        }
        n71 = call "ZenPlusOP600_refaire.vi"("image"="Refaire", "Refaire"=w177, "Cas ok"=OP600ZP_state."Softs" ("casOK"), "errin"=w180, "test ok ?"=w174) -> ("errout"=w175:errorcluster, "Next"=w176:T4)  [unwired: 5 in]
      }
      frame "Conti" {
        # "Continuité des modules pour proto"
        n72 = call "Multi_OUI_NON.vi"("errin"=w205, "errinb"=TRUE, "Tableau"=string[] ["ETIQ", "CONTEST"]) -> ("errout"=w202:errorcluster, "isok?"=w203:bool)  [unwired: 7 in]
        n73 = local write "TOP"("Mesure de continuité" ("TOP")) -> ()
        n74 = case shown="True" w203 {
          selector: w203 -> [w228 _]
          tunnel: w202 -> [w229 w237]
          tunnel: [w229 w233] -> w209
          tunnel: [w228 w235] -> w215
          tunnel: ["0" w231] -> w211
          tunnel: ["ERR" w231] -> w210
          frame False {
          }
          frame True {
            w236 = i16 2 ("largeur (-)")
            n75 = call "Ground Continuity"("Enable"=TRUE, "error in (no error)"=w237) -> ("Conti"=w232:dbl, "error out"=w233:errorcluster)  [unwired: 15 in, 1 out]
            n76 = global read "OP600ZP_VGConf.vi" "Rmax"() -> (w230:dbl)
            n77 = Less Or Equal?(x=w232, y=w230) -> (x <= y?=w235:bool)
            n78 = Number To Fractional String(number=w232, width (-)=w236, precision (6)=w236) -> (F-format string=w231:string)  [unwired: 1 in]
          }
        }
        n79 = local read "Cluster"() -> (w213:T1)
        n80 = Concatenate Strings("Conti;" ("chaîne"), w210) -> (w225:string)
        n81 = Bundle By Name(cluster=w213, "Conti"=w211) -> (w212:T1)
        n82 = call <userlib>:"Log_basic.vi"("errin"=w223, "date?"=TRUE, "chaîne"=w225, "in"=w222) -> ("sortie d'erreur"=w220:errorcluster, "refnum en sortie"=w221:refnum<file>)  [unwired: 6 in]
        n83 = call "ZenPlusOP600_refaire.vi"("image"="Refaire", "Refaire"=w207, "Cas ok"=OP600ZP_state."CAN Resistance" ("casOK"), "errin"=w209, "test ok ?"=w215) -> ("errout"=w216:errorcluster, "Next"=w206:T4)  [unwired: 5 in]
        n84 = local write "Cluster"(w212) -> ()
      }
      frame "CAN Resistance" {
        n85 = call "OUINON.vi"("errin"=w263, "image"="CANRES" ("IN")) -> ("error out"=w262:errorcluster, "OUI/NON"=w261:bool)  [unwired: 8 in]
        n86 = call "Impédance2"("Enable"=w261, "error in (no error)"=w262) -> ("Résistance CAN_BAT / CAN DIAG"=w252:dbl, "Résistance CAN_VEH / CAN SYS"=w256:dbl, "OK"=w258:bool, "error out"=w259:errorcluster)  [unwired: 14 in]
        n87 = Number To Fractional String(number=w256, precision (6)=i16 2 ("précision (6)")) -> (F-format string=w254:string)  [unwired: 2 in]
        n88 = Number To Fractional String(number=w252, precision (6)=i16 2 ("précision (6)")) -> (F-format string=w251:string)  [unwired: 2 in]
        n89 = call "ZenPlusOP600_refaire.vi"("image"="Refaire", "Refaire"=w242, "Cas ok"=OP600ZP_state."VAT" ("casOK"), "errin"=w259, "test ok ?"=w258) -> ("errout"=w239:errorcluster, "Next"=w240:T4)  [unwired: 5 in]
        n90 = Concatenate Strings("CAN Resistance;" ("chaîne"), "CAN_VEH / CAN_SYS;" ("chaîne"), w254, ";CAN_BAT / CAN_DIAG;" ("chaîne"), w251) -> (w249:string)
        n91 = call <userlib>:"Log_basic.vi"("errin"=w248, "date?"=TRUE, "chaîne"=w249, "in"=w246) -> ("sortie d'erreur"=w247:errorcluster, "refnum en sortie"=w245:refnum<file>)  [unwired: 6 in]
      }
      frame "Softs" {
        # "\"C:\\Users\\Operateur\\Desktop\\FORSEE Diag tool V1.7.1\\FORSEE_Diag.exe\""
        # "A réactiver lorsque license sur poste"
        # "C:\\Users\\operateur\\Desktop\\synchro_GENII.bat"
        # "Lancement ForseeDiag Tool"
        # "Injection des softs (ASW, CONFIG, ASW, APPLI)"
        n92 = local write "TOP"("Injection des Softwares" ("TOP")) -> ()
        n93 = disable-structure shown="Désactivé" {
          disable-tunnel: [w285 w287] -> w269
          disable-tunnel: w266 -> [w284 w287]
          frame Disabled {
            # "lancement Synchro_GENII"
            n94 = call "OP600ZP_LaunchEXE.vi"("errin"=w284) -> ("error out"=w286:errorcluster)  [unwired: 8 in]
            n95 = call "OP600ZP_Softs.vi"("errin"=w286) -> ("errout"=w285:errorcluster)  [unwired: 9 in, 1 out]
          }
          frame Enabled {
          }
        }
        n96 = call "OUINON.vi"("errin"=w269, "image"="ALIMON") -> ("error out"=w268:errorcluster, "OUI/NON"=w270:bool)  [unwired: 8 in]
        n97 = call "OP600ZP_LaunchEXE.vi"("errin"=w268, "Application à lancer"=path "C:/Users/Operateur/Desktop/FORSEE Diag tool V1.7.1/FORSEE_Diag.exe") -> ("error out"=w279:errorcluster)  [unwired: 7 in]
        n98 = call "Multi_OUI_NON.vi"("errin"=w279, "errinb"=w270, "Tableau"=string[] ["FDTCHECK", "FDTDTC1"]) -> ("errout"=w276:errorcluster, "isok?"=w274:bool)  [unwired: 7 in]
        n99 = call "ZenPlusOP600_refaire.vi"("image"="Refaire", "Refaire"=w273, "Cas ok"=OP600ZP_state."MCU" ("casOK"), "errin"=w276, "test ok ?"=w274) -> ("errout"=w275:errorcluster, "Next"=w271:T4)  [unwired: 5 in]
      }
      frame "MCU" {
        n100 = local write "TOP"("Mesure MCU" ("TOP")) -> ()
        n101 = call "OUINON.vi"("errin"=w294, "image"="TEMPU") -> ("error out"=w293:errorcluster, "OUI/NON"=w292:bool)  [unwired: 8 in]
        n102 = case shown="True" w292 {
          tunnel: ["" ("Log") w316] -> w297
          tunnel: [w308 w311] -> w298
          tunnel: [FALSE ("is OK?") w315] -> w288
          tunnel: w293 -> [w308 w312]
          frame False {
          }
          frame True {
            n103 = call "OUINON.vi"("errin"=w312, "image"="DATAFDT") -> ("error out"=w313:errorcluster)  [unwired: 8 in, 1 out]
            n104 = call "OP600ZP_FDT_V2.vi"("errin"=w313) -> ("errout"=w311:errorcluster, "Log"=w316:string, "is OK?"=w315:bool)  [unwired: 8 in]
          }
        }
        n105 = Concatenate Strings(w297) -> (w296:string)
        n106 = call <userlib>:"Log_basic.vi"("errin"=w306, "date?"=TRUE, "chaîne"=w296, "in"=w305) -> ("sortie d'erreur"=w304:errorcluster, "refnum en sortie"=w303:refnum<file>)  [unwired: 6 in]
        n107 = call "ZenPlusOP600_refaire.vi"("image"="Refaire", "Refaire"=w291, "Cas ok"=OP600ZP_state."Iso" ("Énum"), "errin"=w298, "test ok ?"=w288) -> ("errout"=w299:errorcluster, "Next"=w289:T4)  [unwired: 5 in]
      }
      frame "Iso" {
        # "test d'isolement PDU+, PDU-, bat+et Bat-"
        n108 = call "OUINON.vi"("errin"=w320, "image"="ISOP" ("IN")) -> ("error out"=w328:errorcluster, "OUI/NON"=w327:bool)  [unwired: 8 in]
        n109 = local write "TOP"("Test d'isolement du Pack" ("TOP")) -> ()
        n110 = control-ref of="TOP"() -> (w329:refnum<vi>)
        n111 = control-ref of="Cluster"() -> (w330:refnum<vi>)
        n112 = call "OP600ZP_ISO.vi"("entrée d'erreur (pas d'erreur)"=w328, "Oui"=w327, "reference en entrée"=w329, "Cluster en entrée"=w330) -> ("sortie d'erreur"=w325:errorcluster, "Chaîne 2"=w333:string, "Chaîne"=w331:string, "Booléen"=w323:bool)  [unwired: 4 in]
        n113 = Concatenate Strings("Iso+;" ("chaîne"), w331, ";Iso-;" ("chaîne"), w333) -> (w332:string)
        n114 = call "ZenPlusOP600_refaire.vi"("image"="Refaire", "Refaire"=w319, "Cas ok"=OP600ZP_state."OCV" ("casOK"), "errin"=w325, "test ok ?"=w323) -> ("errout"=w324:errorcluster, "Next"=w317:T4)  [unwired: 5 in]
        n115 = call <userlib>:"Log_basic.vi"("errin"=w339, "date?"=TRUE, "chaîne"=w332, "in"=w338) -> ("sortie d'erreur"=w340:errorcluster, "refnum en sortie"=w337:refnum<file>)  [unwired: 6 in]
      }
      frame "OCV" {
        # "Ratio Ubatt/OCV critère"
        # "OCV critère"
        # "Test OVC et ACIR"
        n116 = call <userlib>:"FGV_Image.vi"("Énum"=FGV."SET", "IN"="OCV") -> ()  [unwired: 9 in, 1 out]
        n117 = call "Mesure OCV"("Enable"=TRUE, "error in (no error)"=w364) -> ("Tension Bat+ Bat- (V)"=w343:dbl, "error out"=w354:errorcluster)  [unwired: 15 in, 1 out]
        n118 = local write "TOP"("Meusure de la tension à vide" ("TOP")) -> ()
        n119 = global read "Ubatt.vi" "Ubatt"() -> (w350:dbl)
        n120 = global write "OCV.vi" "OCV"(w343) -> ()
        n121 = expression code="x+0.02*x"(w350) -> (w357:dbl)
        n122 = expression code="x-0.02*x"(w350) -> (w358:dbl)
        n123 = call <userlib>:"GetP.vi"("errin"=w354, "Pédale ON?"=FALSE) -> ("errout"=w352:errorcluster)  [unwired: 8 in, 1 out]
        n124 = Max & Min(x=w350, y=w343) -> (max(x,y)=w349:dbl, min(x,y)=w348:dbl)
        n125 = In Range and Coerce(upper limit=w357, x=w343, lower limit=w358) -> (In Range?=w356:bool)  [unwired: 1 out]
        n126 = global read "OP600ZP_VGConf.vi" "RatioUBATTOCV"() -> (w351:dbl)
        n127 = Divide(x=w349, y=w348) -> (x/y=w342:dbl)
        n128 = Less Or Equal?(x=w342, y=w351) -> (x <= y?=w347:bool)
        n129 = Compound Arithmetic op=AND ("Opérateur arithmétique")(w356, w347) -> (w355:bool)
        n130 = case shown="True" w355 {
          tunnel: [w373 w386] -> w361
          tunnel: w343 -> [_ w385]
          tunnel: ["0" w384] -> w365
          tunnel: w362 -> [w373 w383]
          tunnel: w360 -> [w374 w382]
          tunnel: [w374 w381] -> w359
          tunnel: w342 -> [_ w376]
          frame False {
          }
          frame True {
            n131 = Number To Decimal String(number=w385, width (-)=i16 2 ("largeur (-)")) -> (decimal integer string=w384:string)
            n132 = Number To Decimal String(number=w376, width (-)=i16 2 ("largeur (-)")) -> (decimal integer string=w379:string)
            n133 = Concatenate Strings("OCV;" ("chaîne"), w384, ";Ratio OCV/Ubatt;" ("chaîne"), w379) -> (w388:string)
            n134 = call <userlib>:"Log_basic.vi"("errin"=w382, "date?"=TRUE, "chaîne"=w388, "in"=w383) -> ("sortie d'erreur"=w381:errorcluster, "refnum en sortie"=w386:refnum<file>)  [unwired: 6 in]
          }
        }
        n135 = local read "Cluster"() -> (w367:T1)
        n136 = Bundle By Name(cluster=w367, "OCV"=w365) -> (w366:T1)
        n137 = call "ZenPlusOP600_refaire.vi"("image"="Refaire", "Refaire"=w346, "Cas ok"=OP600ZP_state."DTC" ("Énum"), "errin"=w352, "test ok ?"=w355) -> ("errout"=w363:errorcluster, "Next"=w344:T4)  [unwired: 5 in]
        n138 = local write "Cluster"(w366) -> ()
      }
      frame "DTC" {
        # "Chercher moyen de simplifier"
        # "Vérification de l'absence de DTC dans FDT"
        n139 = call "OUINON.vi"("errin"=w400, "image"="DTC1" ("IN")) -> ("error out"=w414:errorcluster, "OUI/NON"=w415:bool)  [unwired: 8 in]
        n140 = case shown="True" w415 {
          tunnel: w414 -> [w433 w439]
          tunnel: [w433 w436] -> w399
          tunnel: [w432 w437] -> w398
          tunnel: [w432 w435] -> w394
          tunnel: [w432 w434] -> w395
          frame False {
            w432 = FALSE ("Aucun DTC")
          }
          frame True {
            n141 = call "Boîte de dialogue utilisateur"("Enable"=TRUE, "error in (no error)"=w439) -> ("Présence de DTC"=w434:bool, "Aucun DTC"=w435:bool, "OK"=w437:bool, "error out"=w436:errorcluster)  [unwired: 14 in]
          }
        }
        n142 = local write "TOP"("Vérification absence DTC" ("TOP")) -> ()
        n143 = And(x=w398, y=w394) -> (x .and. y?=w396:bool)
        n144 = case shown="True" w396 {
          selector: w396 -> [_ w422]
          tunnel: [w417 w421] -> w397
          tunnel: w395 -> [w418 w423]
          frame False {
            n145 = case shown="False" w418 {
              tunnel: [FALSE FALSE] -> w417
              frame False {
              }
              frame True {
              }
            }
          }
          frame True {
            n146 = case shown="True" w423 {
              tunnel: w422 -> [w424 _]
              tunnel: [w424 FALSE] -> w421
              frame False {
              }
              frame True {
              }
            }
          }
        }
        n147 = case shown="True" w397 {
          selector: w397 -> [w427 w431]
          tunnel: w399 -> [w428 w429]
          tunnel: [w428 w429] -> w412
          tunnel: [w427 w431] -> w410
          tunnel: [";DTC DETECTE(S)" "NO DTC;"] -> w402
          frame False {
          }
          frame True {
          }
        }
        n148 = Concatenate Strings("DTC;" ("chaîne"), w402) -> (w409:string)
        n149 = call <userlib>:"Log_basic.vi"("errin"=w406, "date?"=TRUE, "chaîne"=w409, "in"=w404) -> ("sortie d'erreur"=w405:errorcluster, "refnum en sortie"=w403:refnum<file>)  [unwired: 6 in]
        n150 = call "ZenPlusOP600_refaire.vi"("image"="Refaire", "Refaire"=w393, "Cas ok"=OP600ZP_state."Capacitance" ("casOK"), "errin"=w412, "test ok ?"=w410) -> ("errout"=w411:errorcluster, "Next"=w391:T4)  [unwired: 5 in]
      }
      frame "Capacitance" {
        w444 = 1000.0 ("y")
        w469 = i16 2 ("précision (6)")
        # "Valeur lue MX5060 en uF"
        n151 = call "OUINON.vi"("errin"=w483, "image"="CAPA1" ("IN")) -> ("error out"=w482:errorcluster, "OUI/NON"=w478:bool)  [unwired: 8 in]
        n152 = case shown="True" w478 {
          tunnel: w482 -> [w495 w500]
          tunnel: [w495 w497] -> w480
          tunnel: [FALSE ("Aucun DTC") w498] -> _
          tunnel: [0.0 ("Valeur de la capacité BAT+") w496] -> w445
          frame False {
          }
          frame True {
            n153 = call "Mesure de capacité BAT+"("Enable"=TRUE, "error in (no error)"=w500) -> ("Valeur de la capacité BAT+"=w496:dbl, "OK"=w498:bool, "error out"=w497:errorcluster)  [unwired: 15 in]
          }
        }
        n154 = local write "TOP"("Test de capacité" ("TOP")) -> ()
        n155 = call "OUINON.vi"("errin"=w480, "image"="CAPA2" ("IN")) -> ("error out"=w479:errorcluster, "OUI/NON"=w477:bool)  [unwired: 8 in]
        n156 = case shown="True" w477 {
          tunnel: w479 -> [w487 w492]
          tunnel: [w487 w489] -> w463
          tunnel: [FALSE ("Aucun DTC") w490] -> _
          tunnel: [0.0 ("Valeur de la capacité BAT-") w488] -> w447
          frame False {
          }
          frame True {
            n157 = call "Mesure de capacité BAT-"("Enable"=TRUE, "error in (no error)"=w492) -> ("Valeur de la capacité BAT-"=w488:dbl, "OK"=w490:bool, "error out"=w489:errorcluster)  [unwired: 15 in]
          }
        }
        n158 = global read "OP600ZP_VGConf.vi" "CBAT+"() -> (w450:dbl)
        n159 = global read "OP600ZP_VGConf.vi" "CBAT-"() -> (w453:dbl)
        n160 = Divide(x=w453, y=1000.0) -> (x/y=w452:dbl)
        n161 = Multiply(x=w447, y=w444) -> (x*y=w446:dbl)
        n162 = Multiply(x=w445, y=w444) -> (x*y=w443:dbl)
        n163 = global read "OP600ZP_VGConf.vi" "CBATmin"() -> (w441:dbl)
        n164 = Divide(x=w450, y=1000.0) -> (x/y=w448:dbl)
        n165 = Number To Fractional String(number=w446, precision (6)=w469) -> (F-format string=w466:string)  [unwired: 2 in]
        n166 = Number To Fractional String(number=w443, precision (6)=w469) -> (F-format string=w467:string)  [unwired: 2 in]
        n167 = Divide(x=w441, y=1000.0) -> (x/y=w440:dbl)
        n168 = In Range and Coerce(upper limit=w452, x=w447, lower limit=w440) -> (In Range?=w455:bool)  [unwired: 1 out]
        n169 = In Range and Coerce(upper limit=w448, x=w445, lower limit=w440) -> (In Range?=w454:bool)  [unwired: 1 out]
        n170 = And(x=w455, y=w454) -> (x .and. y?=w462:bool)
        n171 = Concatenate Strings("Capacitance;" ("chaîne"), "CBAT+;" ("chaîne"), w467, ";CBAT-;" ("chaîne"), w466) -> (w471:string)
        n172 = call "ZenPlusOP600_refaire.vi"("image"="Refaire", "Refaire"=w460, "Cas ok"=OP600ZP_state."INTERLOOP" ("casOK"), "errin"=w463, "test ok ?"=w462) -> ("errout"=w461:errorcluster, "Next"=w458:T4)  [unwired: 5 in]
        n173 = call <userlib>:"Log_basic.vi"("errin"=w475, "date?"=TRUE, "chaîne"=w471, "in"=w473) -> ("sortie d'erreur"=w474:errorcluster, "refnum en sortie"=w472:refnum<file>)  [unwired: 6 in]
      }
      frame "INTERLOOP" {
        # "111111"
        n174 = local write "TOP"("Test Interlock Loop" ("TOP")) -> ()
        n175 = call "OUINON.vi"("errin"=w508, "image"="DTC_DRIVE") -> ("error out"=w506:errorcluster, "OUI/NON"=w505:bool)  [unwired: 8 in]
        n176 = call "DTC DRIVE"("Enable"=w505, "error in (no error)"=w506) -> ("Absence de DTC?"=w502:bool, "error out"=w504:errorcluster)  [unwired: 15 in, 1 out]
        n177 = call "OP600ZP_INTLCK_LOOP.vi"("entrée d'erreur (pas d'erreur)"=w504) -> ("sortie d'erreur"=w524:errorcluster, "Chaîne 2"=w515:string, "Chaîne 3"=w517:string, "Case à cocher"=w510:bool, "Chaîne"=w513:string, "cas vrai"=w511:string)  [unwired: 5 in]
        n178 = case shown="True" w502 {
          tunnel: ["DTC" "NO DTC"] -> w501
          frame False {
          }
          frame True {
          }
        }
        n179 = Concatenate Strings("INTERLOOP;" ("chaîne"), "X & Y débranchés;" ("chaîne"), w517, ";Y débranché;" ("chaîne"), w515, ";X débranché;" ("chaîne"), w513, ";X & Y branchés;" ("chaîne"), w511, ";DTC DRIVE;" ("chaîne"), w501) -> (w531:string)
        n180 = call <userlib>:"Log_basic.vi"("errin"=w529, "date?"=TRUE, "chaîne"=w531, "in"=w530) -> ("sortie d'erreur"=w528:errorcluster, "refnum en sortie"=w527:refnum<file>)  [unwired: 6 in]
        n181 = call "ZenPlusOP600_refaire.vi"("image"="Refaire", "Refaire"=w523, "Cas ok"=OP600ZP_state."PreCharge" ("casOK"), "errin"=w524, "test ok ?"=w510) -> ("errout"=w521:errorcluster, "Next"=w522:T4)  [unwired: 5 in]
      }
      frame "Current + DCIR" {
        n182 = call "OUINON.vi"("errin"=w577, "image"="DCIR1" ("IN")) -> ("error out"=w575:errorcluster, "OUI/NON"=w576:bool)  [unwired: 8 in]
        n183 = case shown="True" w576 {
          tunnel: w575 -> [w618 w625]
          tunnel: [w618 w623] -> w548
          tunnel: [w617 w621] -> w556
          tunnel: [w617 w620] -> w555
          tunnel: [w617 w619] -> w554
          frame False {
            w617 = 1000.0 ("Battery Current")
          }
          frame True {
            n184 = call "OUINON.vi"("errin"=w625, "image"="DCIR2" ("IN")) -> ("error out"=w624:errorcluster, "OUI/NON"=w622:bool)  [unwired: 8 in]
            n185 = call "ZeroCurrent"("Enable"=w622, "error in (no error)"=w624) -> ("DeltaT@0s"=w619:dbl, "DeltaV@0s"=w620:dbl, "BatteryCurrent"=w621:dbl, "error out"=w623:errorcluster)  [unwired: 13 in, 1 out]
          }
        }
        n186 = local write "TOP"("Test DCIR" ("TOP")) -> ()
        n187 = call <vilib>:"System Exec.vi"("run minimized? (F)"=TRUE, "wait until completion? (T)"=FALSE, "error in (no error)"=w548, "working directory"=path "C:/Program Files ", "command line"="cmd /c start WindowsApps\\Microsoft.ScreenSketch_11.2303.17.0_x64__8wekyb3d8bbwe\\SnippingTool\\SnippingTool.exe") -> ()  [unwired: 3 in, 4 out]
        n188 = call "OUINON.vi"("errin"=w548, "image"="DCIR3") -> ("error out"=w573:errorcluster, "OUI/NON"=w572:bool)  [unwired: 8 in]
        n189 = case shown="True" w572 {
          tunnel: w573 -> [w602 w615]
          tunnel: [w602 w603] -> w542
          tunnel: [FALSE ("OK") w614] -> w540
          tunnel: [0.0 ("Battery Voltage") w613] -> w560
          tunnel: [0.0 ("Battery Current") w612] -> w559
          tunnel: [0.0 ("DeltaVoltage") w611] -> w558
          tunnel: [0.0 ("DeltaTemp") w610] -> w557
          frame False {
          }
          frame True {
            n190 = call "OUINON.vi"("errin"=w615, "image"="DCIR4") -> ("error out"=w609:errorcluster, "OUI/NON"=w608:bool)  [unwired: 8 in]
            n191 = call "Voltage /Current / Temp"("Enable"=w608, "error in (no error)"=w609) -> ("DeltaT@30s"=w610:dbl, "DeltaV@30s"=w611:dbl, "BatteryCurrent@30s"=w612:dbl, "BatteryVoltage@30s"=w613:dbl, "OK"=w614:bool, "error out"=w603:errorcluster)  [unwired: 12 in]
            n192 = call <vilib>:"System Exec.vi"("run minimized? (F)"=TRUE, "wait until completion? (T)"=FALSE, "error in (no error)"=w603, "working directory"=path "C:/Program Files ", "command line"="cmd /c Taskkill/PID SnippingTool.exe /F") -> ()  [unwired: 3 in, 4 out]
          }
        }
        n193 = call "OUINON.vi"("errin"=w542, "image"="JAUGE") -> ("error out"=w541:errorcluster, "OUI/NON"=w539:bool)  [unwired: 8 in]
        n194 = And(x=w539, y=w540) -> (x .and. y?=w538:bool)
        n195 = case shown="True" w538 {
          tunnel: w541 -> [w581 w582]
          tunnel: [w581 w588] -> w545
          tunnel: [FALSE ("OK") w586] -> w537
          tunnel: [0.0 ("Post Relax Voltage :") w587] -> w544
          frame False {
          }
          frame True {
            n196 = while {
              tunnel: [w594] -> w584
              tunnel: w582 -> [w593]
              tunnel: [w593] -> w592
              stop <- w594 stop-if-true
              n197 = global read "VG_progressBar.vi" "progression"() -> (w596:dbl)
              "Progres" <- w596
              n198 = Equal?(x=w596, y=u8 0) -> (x = y?=w594:bool)
            }
            n199 = call "Timer2.vi"("error out"=w582) -> ("errout"=w591:errorcluster, "30s?"=w585:bool)  [unwired: 9 in]
            n200 = And(x=w585, y=w584) -> (x .and. y?=w583:bool)
            n201 = Merge Errors(w591, w592) -> (w590:errorcluster)
            n202 = call "Post Relax"("Enable"=w583, "error in (no error)"=w590) -> ("Post Relax Voltage :"=w587:dbl, "error out"=w589:errorcluster)  [unwired: 15 in, 1 out]
            n203 = call "OP600ZP_Ubatt_Post_Relax.vi"("errin"=w589, "Ubatt Post Relax"=w587) -> ("errout"=w588:errorcluster, "Dans la gamme ?"=w586:bool)  [unwired: 6 in, 2 out]
          }
        }
        n204 = Bundle("BatteryVoltage@30s"=w560, "BatteryCurrent@30s"=w559, "DeltaV@30s"=w558, "DeltaT@30s"=w557, "BatteryCurrent"=w556, "DeltaV@0s"=w555, "DeltaT@0s"=w554, "Post Relax Voltage :"=w544) -> (w553:T6)  [unwired: 1 in]
        n205 = call "OP600ZP_Assembly.vi"("DCIR_MESURES"=w553) -> ("Out"=w552:string, "PASS/FAIL"=w536:bool)  [unwired: 8 in]
        n206 = And(x=w537, y=w536) -> (x .and. y?=w535:bool)
        n207 = call <userlib>:"Log_basic.vi"("errin"=w564, "date?"=TRUE, "chaîne"=w552, "in"=w562) -> ("sortie d'erreur"=w563:errorcluster, "refnum en sortie"=w561:refnum<file>)  [unwired: 6 in]
        n208 = call "ZenPlusOP600_refaire.vi"("image"="Refaire", "Refaire"=w569, "Cas ok"=OP600ZP_state."DTC2" ("casOK"), "errin"=w545, "test ok ?"=w535) -> ("errout"=w570:errorcluster, "Next"=w566:T4)  [unwired: 5 in]
      }
      frame "PreCharge" {
        w658 = 5.0 ("x")
        # "Voir Quentin car test plan va tout NOK\nATTENTION A MODIFIER AUSSI DANS PV GENERATOR"
        n209 = call "Multi_OUI_NON.vi"("errin"=w665, "errinb"=TRUE, "Tableau"=string[] ["PRECHARGE1", "PRECHARGE2", "PRE_FUSE"]) -> ("errout"=w640:errorcluster, "isok?"=w641:bool)  [unwired: 7 in]
        n210 = call "PRE_FUSE"("Enable"=w641, "error in (no error)"=w640) -> ("OK"=w642:bool, "error out"=w662:errorcluster)  [unwired: 15 in, 1 out]
        n211 = case shown="True" w642 {
          tunnel: w662 -> [w678 w684]
          tunnel: [w678 w680] -> w661
          tunnel: [FALSE ("OK") w679] -> w635
          frame False {
            (unwired) 0.0 ("Tension")
          }
          frame True {
            n212 = call "OUINON.vi"("errin"=w684, "image"="PRECHARGE3") -> ("error out"=w681:errorcluster, "OUI/NON"=w682:bool)  [unwired: 8 in]
            n213 = call "Tension"("Enable"=w682, "error in (no error)"=w681) -> ("OK"=w679:bool, "error out"=w680:errorcluster)  [unwired: 15 in, 1 out]
          }
        }
        n214 = local write "TOP"("Precharge" ("TOP")) -> ()
        n215 = case shown="True" w635 {
          tunnel: w661 -> [w669 w673]
          tunnel: [w669 w672] -> w629
          tunnel: [0.0 ("Final Voltage :") w671] -> w636
          tunnel: [FALSE ("OK") w670] -> w632
          frame False {
          }
          frame True {
            n216 = call "OUINON.vi"("errin"=w673, "image"="PRECHARGE4") -> ("error out"=w676:errorcluster, "OUI/NON"=w675:bool)  [unwired: 8 in]
            n217 = call "Final Voltage"("Enable"=w675, "error in (no error)"=w676) -> ("Final Voltage :"=w671:dbl, "OK"=w670:bool, "error out"=w672:errorcluster)  [unwired: 15 in]
          }
        }
        n218 = global read "OCV.vi" "OCV"() -> (w659:dbl)
        n219 = Add(x=w658, y=w659) -> (x+y=w660:dbl)
        n220 = Subtract(x=w659, y=w658) -> (x-y=w657:dbl)
        n221 = In Range and Coerce(upper limit=w660, x=w636, lower limit=w657) -> (coerced(x)=w652:dbl, In Range?=w639:bool)
        n222 = And(x=w632, y=w639) -> (x .and. y?=w630:bool)
        n223 = call "Multi_OUI_NON.vi"("errin"=w629, "errinb"=w630, "Tableau"=string[] ["PRECHARGE5", "CAPAOUT"]) -> ("errout"=w627:errorcluster, "isok?"=w628:bool)  [unwired: 7 in]
        n224 = Number To Fractional String(number=w652, precision (6)=i16 2 ("précision (6)")) -> (F-format string=w654:string)  [unwired: 2 in]
        n225 = Concatenate Strings("PreCharge;" ("chaîne"), "VBatterie;" ("chaîne"), ";FinalVoltage;" ("chaîne"), w654) -> (w655:string)
        n226 = call <userlib>:"Log_basic.vi"("errin"=w648, "date?"=TRUE, "chaîne"=w655, "in"=w651) -> ("sortie d'erreur"=w649:errorcluster, "refnum en sortie"=w650:refnum<file>)  [unwired: 6 in]
        n227 = call "ZenPlusOP600_refaire.vi"("image"="Refaire", "Refaire"=w644, "Cas ok"=OP600ZP_state."Current + DCIR" ("casOK"), "errin"=w627, "test ok ?"=w628) -> ("errout"=w645:errorcluster, "Next"=w643:T4)  [unwired: 5 in]
      }
      frame "DTC2" {
        # "Chercher moyen de simplifier"
        n228 = call "OUINON.vi"("errin"=w697, "image"="DTC1" ("IN")) -> ("error out"=w711:errorcluster, "OUI/NON"=w712:bool)  [unwired: 8 in]
        n229 = local write "TOP"("Vérification absence DTC n°2" ("TOP")) -> ()
        n230 = case shown="True" w712 {
          tunnel: w711 -> [w736 w742]
          tunnel: [w736 w739] -> w705
          tunnel: [w735 w740] -> w704
          tunnel: [w735 w738] -> w700
          tunnel: [w735 w737] -> w701
          frame False {
            w735 = FALSE ("Aucun DTC")
          }
          frame True {
            n231 = call "Boîte de dialogue utilisateur2"("Enable"=TRUE, "error in (no error)"=w742) -> ("Présence de DTC"=w737:bool, "Aucun DTC"=w738:bool, "OK"=w740:bool, "error out"=w739:errorcluster)  [unwired: 14 in]
          }
        }
        n232 = And(x=w704, y=w700) -> (x .and. y?=w702:bool)
        n233 = case shown="True" w702 {
          selector: w702 -> [_ w725]
          tunnel: [w720 w724] -> w703
          tunnel: w701 -> [w721 w726]
          frame False {
            n234 = case shown="False" w721 {
              tunnel: [FALSE FALSE] -> w720
              frame False {
              }
              frame True {
              }
            }
          }
          frame True {
            n235 = case shown="True" w726 {
              tunnel: w725 -> [w727 _]
              tunnel: [w727 FALSE] -> w724
              frame False {
              }
              frame True {
              }
            }
          }
        }
        n236 = case shown="True" w703 {
          selector: w703 -> [w730 w734]
          tunnel: w705 -> [w731 w732]
          tunnel: [w731 w732] -> w686
          tunnel: [w730 w734] -> w685
          tunnel: [";DTC DETECTE(S)" "NO DTC;"] -> w706
          frame False {
          }
          frame True {
          }
        }
        n237 = Concatenate Strings("DTC2;" ("chaîne"), w706) -> (w709:string)
        n238 = call <userlib>:"Log_basic.vi"("errin"=w695, "date?"=TRUE, "chaîne"=w709, "in"=w696) -> ("sortie d'erreur"=w692:errorcluster, "refnum en sortie"=w693:refnum<file>)  [unwired: 6 in]
        n239 = case shown="True" w685 {
          tunnel: w686 -> [w714 w718]
          tunnel: [w714 w717] -> w688
          tunnel: [FALSE ("OUI/NON") w716] -> w687
          frame False {
          }
          frame True {
            n240 = call "OUINON.vi"("errin"=w718, "image"="VAT3" ("IN")) -> ("error out"=w717:errorcluster, "OUI/NON"=w716:bool)  [unwired: 8 in]
          }
        }
        n241 = call "ZenPlusOP600_refaire.vi"("image"="Refaire", "Refaire"=w698, "Cas ok"=OP600ZP_state."PARK" ("casOK"), "errin"=w688, "test ok ?"=w687) -> ("errout"=w689:errorcluster, "Next"=w691:T4)  [unwired: 5 in]
      }
      frame "PARK" {
        n242 = call "OUINON.vi"("errin"=w750, "image"="POST_FUSE") -> ("error out"=w745:errorcluster, "OUI/NON"=w744:bool)  [unwired: 8 in]
        n243 = local write "TOP"("Mesure MCU PARK" ("TOP")) -> ()
        n244 = call "Poste_Fuse"("Enable"=w744, "error in (no error)"=w745) -> ("OK"=w748:bool, "error out"=w749:errorcluster)  [unwired: 15 in, 1 out]
        n245 = case shown="True" w748 {
          tunnel: [w764 w766] -> w752
          tunnel: w749 -> [w764 w765]
          frame False {
          }
          frame True {
            n246 = call "OUINON.vi"("errin"=w765, "image"="DATAFDT2") -> ("error out"=w766:errorcluster)  [unwired: 8 in, 1 out]
          }
        }
        n247 = call "OP600ZP_FDT_FIN.vi"("errin"=w752) -> ("errout"=w747:errorcluster, "Log"=w743:string, "is OK?"=w751:bool)  [unwired: 8 in]
        n248 = call "ZenPlusOP600_refaire.vi"("image"="Refaire", "Refaire"=w759, "Cas ok"=OP600ZP_state."FIN_TEST" ("Énum"), "errin"=w747, "test ok ?"=w751) -> ("Next"=w758:T4)  [unwired: 5 in, 1 out]
        n249 = call <userlib>:"Log_basic.vi"("errin"=w757, "date?"=TRUE, "chaîne"=w743, "in"=w756) -> ("sortie d'erreur"=w754:errorcluster, "refnum en sortie"=w753:refnum<file>)  [unwired: 6 in]
      }
      frame "FIN_TEST" {
        n250 = local write "TOP"("Fin de test" ("TOP")) -> ()
        n251 = call "Multi_OUI_NON.vi"("errin"=w772, "errinb"=TRUE, "Tableau"=string[] ["ETIQ2", "END1", "END2", "END3", "END4", "END5"]) -> ("errout"=w777:errorcluster, "isok?"=w776:bool)  [unwired: 7 in]
        n252 = case shown="True" w776 {
          tunnel: [w783 w794] -> w770
          tunnel: w771 -> [w783 w793]
          tunnel: [w782 w792] -> w769
          tunnel: w768 -> [w782 w791]
          frame False {
          }
          frame True {
            n253 = Concatenate Strings("FIN_TEST;" ("chaîne"), "ETIQ2;" ("chaîne"), "OK;" ("chaîne"), "Esthetique Pack;" ("chaîne"), "OK;" ("chaîne"), "VAT2;" ("chaîne"), "OK" ("chaîne")) -> (w795:string)
            n254 = call <userlib>:"Log_basic.vi"("errin"=w793, "date?"=TRUE, "chaîne"=w795, "in"=w791) -> ("sortie d'erreur"=w794:errorcluster, "refnum en sortie"=w792:refnum<file>)  [unwired: 6 in]
          }
        }
        n255 = call "ZenPlusOP600_refaire.vi"("image"="Refaire", "Refaire"=w774, "Cas ok"=OP600ZP_state."Next" ("casOK"), "errin"=w777, "test ok ?"=w776) -> ("Next"=w773:T4)  [unwired: 5 in, 1 out]
      }
      frame "Crash" {
        # "\\\\forseepower.com\\fr\\040 Production\\FR7 - Poitiers\\06 Production\\05. Electronique\\Documents Control lib\\Archives\\ZEN PLUS"
        n256 = Close File(refnum=w825, error in=w824) -> (path=w809:path, error out=w817:errorcluster)
        n257 = call <userlib>:"FGV_Image.vi"("Énum"=FGV."SET", "IN"="TeamLeader") -> ()  [unwired: 9 in, 1 out]
        n258 = call <userlib>:"waitXms.vi"("attente (ms)"=u32 500, "errin"=w817) -> ("errout"=w810:errorcluster)  [unwired: 13 in]
        n259 = Read from Text File(file (use dialog)=w809, error in=w810) -> (text=w808:string, error out=w806:errorcluster)  [unwired: 2 in, 2 out]
        n260 = call "OP600ZP_SN_Reader.vi"("Fichier txt"=w808) -> ("SN"=w801:string)  [unwired: 10 in]
        n261 = local read "Cluster"() -> (w803:T1)
        n262 = Unbundle By Name(w803) -> ("PN"=w800:string)
        n263 = Concatenate Strings(w800, "-SN" ("chaîne"), w801) -> (w802:string)
        n264 = call "OP600ZP_NouveauDossier.vi"("entrée d'erreur (pas d'erreur)"=w806, "Nom du repertoire (PN SN)"=w802, "Network before adding a new folder"=path "\\\\forseepower.com\\fr/040 Production/FR7 - Poitiers/06 Production/05. Electronique/Documents Control lib/Archives/ZEN PLUS" ("chemin de la cible (utiliser une boîte de dialogue)")) -> ("sortie d'erreur"=w807:errorcluster, "Network after adding a new folder"=w804:path)  [unwired: 7 in]
        n265 = Copy ("Copier")(8:w807, 10:w804, 11:w809) -> (0:w816:errorcluster)  [unwired: 2 in, 2 out]
        n266 = call "PvgeneratorOP600.vi"("errin"=w816, "network"=w804, "path in"=w809) -> ("sortie d'erreur"=w820:errorcluster, "network out"=w819:path)  [unwired: 5 in, 2 out]
        n267 = Select ("Sélectionner")(t="1", s=FALSE ("sélecteur"), f="0" ("cas faux")) -> (s? t:f=w812:string)
        n268 = call <userlib>:"POP_GOOGLE.vi"("error in"=w820, "chemin"=w819) -> ("error out"=w798:errorcluster)  [unwired: 8 in, 1 out]
        n269 = local read "Cluster"() -> (w815:T1)
        n270 = Bundle By Name(cluster=w815, "Résultat final"=w812) -> ()  [unwired: 1 out]
        n271 = flat-sequence {
          tunnel: [TRUE] -> w826
          tunnel: w798 -> [_]
          frame #0 {
          }
        }
      }
      frame "Next" {
        w853 = OP600ZP_state."Null"  # Énum
        w854 = OP600ZP_state."Scan"  # Énum
        # "RFE -> 0334"
        # "\\\\forseepower.com\\fr\\040 Production\\FR7 - Poitiers\\06 Production\\05. Electronique\\Documents Control lib\\Archives\\ZEN PLUS"
        n272 = Close File(refnum=w856, error in=w855) -> (path=w831:path, error out=w852:errorcluster)
        n273 = call <userlib>:"waitXms.vi"("attente (ms)"=u32 500, "errin"=w852) -> ("errout"=w843:errorcluster)  [unwired: 13 in]
        n274 = Read from Text File(file (use dialog)=w831, error in=w843) -> (text=w841:string, error out=w840:errorcluster)  [unwired: 2 in, 2 out]
        n275 = local read "Cluster"() -> (w836:T1)
        n276 = call "OP600ZP_SN_Reader.vi"("Fichier txt"=w841) -> ("SN"=w833:string)  [unwired: 10 in]
        n277 = Unbundle By Name(w836) -> ("PN"=w835:string)
        n278 = Concatenate Strings(w835, "-SN" ("chaîne"), w833) -> (w832:string)
        n279 = call "OP600ZP_NouveauDossier.vi"("entrée d'erreur (pas d'erreur)"=w840, "Nom du repertoire (PN SN)"=w832, "Network before adding a new folder"=path "\\\\forseepower.com\\fr/040 Production/FR7 - Poitiers/06 Production/05. Electronique/Documents Control lib/Archives/ZEN PLUS" ("chemin de la cible (utiliser une boîte de dialogue)")) -> ("sortie d'erreur"=w839:errorcluster, "Network after adding a new folder"=w837:path)  [unwired: 7 in]
        n280 = call "OUINON.vi"("errin"=w858, "image"="Next" ("IN")) -> ("error out"=w830:errorcluster, "OUI/NON"=w857:bool)  [unwired: 8 in]
        n281 = Copy ("Copier")(8:w839, 10:w837, 11:w831) -> (0:w842:errorcluster)  [unwired: 2 in, 2 out]
        n282 = call "PvgeneratorOP600.vi"("errin"=w842, "network"=w837, "path in"=w831) -> ("sortie d'erreur"=w850:errorcluster, "network out"=w849:path, "tout bon"=w847:bool)  [unwired: 5 in, 1 out]
        n283 = Select ("Sélectionner")(t="1", s=w847, f="0" ("cas faux")) -> (s? t:f=w844:string)
        n284 = local read "Cluster"() -> (w848:T1)
        n285 = Bundle By Name(cluster=w848, "Résultat final"=w844) -> ()  [unwired: 1 out]
        n286 = call <userlib>:"POP_GOOGLE.vi"("error in"=w850, "chemin"=w849) -> ("error out"=w829:errorcluster)  [unwired: 8 in, 1 out]
        n287 = Select(t=w854, s=w857, f=w853) -> (s? t:f=w828:T4)
      }
      frame "Comext" {
        n288 = disable-structure shown="Désactivé" {
          disable-tunnel: w870 -> [w884 _]
          disable-tunnel: w869 -> [w883 _]
          disable-tunnel: [w882 _] -> w868
          disable-tunnel: w867 -> [w881 _]
          disable-tunnel: [w880 _] -> w866
          disable-tunnel: w865 -> [w879 _]
          disable-tunnel: w864 -> [w877 _]
          disable-tunnel: [w875 _] -> w863
          disable-tunnel: w862 -> [w874 _]
          disable-tunnel: [w872 _] -> w861
          disable-tunnel: [w871 _] -> w860
          frame Disabled {
            n289 = call "OUINON.vi"("errin"=w877, "image"="Comext" ("IN")) -> ("error out"=w876:errorcluster, "OUI/NON"=w873:bool)  [unwired: 8 in]
            n290 = case shown="True" w873 {
              tunnel: w884 -> [w889 w902]
              tunnel: w883 -> [w888 w901]
              tunnel: [w888 w900] -> w872
              tunnel: [w889 w899] -> w882
              tunnel: [OP600ZP_state."Crash" ("OUT") w898] -> w871
              tunnel: w881 -> [_ w897]
              tunnel: [w886 w896] -> w880
              tunnel: w879 -> [_ w895]
              tunnel: w876 -> [w886 w894]
              tunnel: [w887 w893] -> w875
              tunnel: w874 -> [w887 w893]
              frame False {
              }
              frame True {
                w890 = OP600ZP_state."Scan"  # Énum
                (unwired) "Comext;" ("testname")
                n291 = local read "PN"() -> (w913:string)
                n292 = call <vilib>:"Application Directory.vi"() -> ("Application Directory"=w915:path)
                n293 = call <userlib>:"Read_Param.vi"("Énum"=enum16{"STR", "DBL", "U32"}."U32", "errin"=w894, 9:w915, "section"="DataDyn", "key"=w913) -> ("error out"=w908:errorcluster, "U32"=w911:u32)  [unwired: 2 in, 3 out]
                n294 = call <userlib>:"FGV_Image.vi"("Énum"=FGV."SET", "IN"="DataDyn") -> ()  [unwired: 9 in, 1 out]
                n295 = property on="progression" class="Slide (strict)"(error in=w908, "Visible"=TRUE, "Value"=u8 0 ("progression")) -> (error out=w907:errorcluster)  [unwired: 1 in, 1 out]
                n296 = call "SCAN CMU.vi"("errin"=w907, "Nb modules"=w911) -> ("errout"=w925:errorcluster, "# température + #tension OK?"=w920:bool, "Vmin"=w924:dbl, "Vmax"=w923:dbl, "Tmin"=w921:dbl, "Tmax"=w922:dbl)  [unwired: 4 out]
                n297 = call "OP500ZP_Test_DataDyn.vi"("Vcell Max (V)"=w923, "MCU"=w920, "Vcell Min (V)"=w924, "appdir"=w895, "errin"=w925, "Température usine (°C)"=21.0, "Tcell Max (°C)"=w922, "Tcell Min (°C)"=w921) -> ("errout"=w919:errorcluster, "datalog"=w927:string, "pass"=w918:bool)  [unwired: 1 out]
                n298 = call <userlib>:"Log_basic.vi"("errin"=w902, "date?"=TRUE, "chaîne"=w927, "in"=w901) -> ("sortie d'erreur"=w899:errorcluster, "refnum en sortie"=w900:refnum<file>)  [unwired: 6 in]
                n299 = call "ZenPlusOP600_refaire.vi"("image"="Refaire", "Refaire"=w897, "Pédale"=FALSE, "Cas ok"=w890, "errin"=w919, "test ok ?"=w918) -> ("errout"=w903:errorcluster, "Next"=w898:T4)  [unwired: 4 in]
                n300 = property on="progression" class="Slide (strict)"(error in=w903, "Visible"=FALSE, "Value"=u8 0 ("progression")) -> (error out=w896:errorcluster)  [unwired: 1 in, 1 out]
              }
            }
          }
          frame Enabled {
          }
        }
      }
    }
    n301 = Wait (ms)(milliseconds to wait=u32 200 ("attente (ms)")) -> ()  [unwired: 1 out]
    n302 = case shown="False" w25 {
      selector: w25 -> [_ w928]
      frame False {
      }
      frame True {
        n303 = local write "STOP"(w928) -> ()
      }
    }
  }
  n304 = while {
    shift-right: [w937] -> _
    shift-left: errorcluster {"status"=FALSE, "code"=0, "source"=""} ("error out") -> [w934]
    stop <- w935 stop-if-true
    # "ici tu mets l'image à jour si besoin"
    n305 = Wait (ms)(milliseconds to wait=u32 100 ("attente (ms)")) -> ()  [unwired: 1 out]
    n306 = call <userlib>:"FGV_Image.vi"("Énum"=FGV."GET") -> ("OUT"=w930:string)  [unwired: 10 in]
    n307 = Not Equal?(x=w930, y="") -> (x != y?=w931:bool)
    n308 = case shown="False" w931 {
      tunnel: [w939 w944] -> w937
      tunnel: w934 -> [w939 w943]
      tunnel: w930 -> [_ w942]
      frame False {
      }
      frame True {
        n309 = call <vilib>:"Application Directory.vi"() -> ("Application Directory"=w947:path)
        n310 = Path To String(path=w947) -> (string=w948:string)
        n311 = Concatenate Strings(w948, "\\Image\\" ("chaîne"), w942, ".jpg" ("chaîne")) -> (w946:string)
        n312 = call <userlib>:"FGV_Image.vi"("Énum"=FGV."RAZ") -> ()  [unwired: 10 in, 1 out]
        n313 = String To Path(string=w946) -> (path=w945:path)
        n314 = call <vilib>:"Read JPEG File.vi"("error in (no error)"=w943, "path to JPEG file"=w945) -> ("error out"=w944:errorcluster, "image data"=w951:T7)  [unwired: 7 in, 1 out]
        n315 = call <vilib>:"Draw Flattened Pixmap.vi"("image data"=w951) -> ("new picture"=w940:picture)  [unwired: 8 in]
        n316 = local write "DRAW"(w940) -> ()
      }
    }
    n317 = global read "VG_progressBar.vi" "progression"() -> (→"progression":dbl)
    n318 = local read "STOP"() -> (w936:bool)
    n319 = Or(x=w937, y=w936) -> (x .or. y?=w935:bool)
  }
  n320 = Merge Errors(w17, w16) -> (→"errout":errorcluster)
  n321 = disable-structure shown="Activé" {
    disable-tunnel: [w952 _] -> _
    frame Disabled {
      n322 = call "Data Dynamiques"() -> ("CMU OK"=w952:bool)  [unwired: 12 in, 7 out]
    }
    frame Enabled {
    }
  }
  "STOP" <- w14
